vi "PECT - Scan.vi"() -> ()   [LabVIEW 2012]
uses:
  <vilib>/DAQmx/write.llb/DAQmx Write (Analog 1D Wfm NChan NSamp).vi
  <vilib>/DAQmx/read.llb/DAQmx Read (Analog 1D DBL 1Chan NSamp).vi
  <vilib>/DAQmx/read.llb/DAQmx Read (Analog Wfm 1Chan NSamp).vi
  <vilib>/Instr/_visa.llb/VISA Configure Serial Port (Instr).vi
  <vilib>/DAQmx/create/channels.llb/DAQmx Create Channel (AI-Voltage-Basic).vi
  <vilib>/DAQmx/configure/timing.llb/DAQmx Timing (Sample Clock).vi
  <vilib>/DAQmx/configure/task.llb/DAQmx Configure Logging (TDMS).vi
  <vilib>/DAQmx/configure/trigger.llb/DAQmx Start Trigger (Digital Edge).vi
  <vilib>/DAQmx/create/channels.llb/DAQmx Create Channel (AO-Voltage-Basic).vi
  <vilib>/DAQmx/miscellaneous.llb/DAQmx Fill In Error Info.vi
  Global_data.vi
  <vilib>/express/express analysis/Spectral/Block/exnSpectralBlock spectral measurements PSD poly.vi
  <vilib>/express/express analysis/Spectral/Block/exnSpectralBlock spectral measurements PSD WFM.vi
  <vilib>/express/express analysis/Spectral/XNode/ExpressSpectralMeasurementsBlockNode.xnode
  <resource>/objmgr/daqmx.rc
  <vilib>/measure/NI_MABase.lvlib
  <vilib>/Platform/NI_3dgraph.lvlib
panel:
  in  "Backward scan":bool
  in  "X-length count":dbl=20.0
  out "No.data":i32
  in  "Save Scan mode":bool caption="Save Process"
  in  "Plot style":i32(ring)=5 items=["cwLine"=1, "cwPoint"=2, "cwLinePoint"=3, "cwHiddenLine"=4, "cwSurface"=5, "cwSurfaceLine"=6, "cwSurfaceNormal"=7, "cwContourLine"=8, "cwSurfaceContour"=9]
  in  "Stop 4":bool
  in  "Forward scan":bool
  in  "ViewMode":i32(ring) items=["cwViewXYPlane", "cwViewXZPlane", "cwViewYZPlane", "cwViewUserDefined"]
  in  "Stop Scan 2":bool
  in  "Emergency Stop":bool
  in  "Stop 3":bool
  in  "Home Y":bool
  in  "Home X":bool
  in  "Back":bool
  in  "Front":bool
  in  "Left":bool
  in  "Right":bool
  in  "Stop Scan":bool
  in  "Move Distance (mm)":dbl=10.0
  in  "Scan":bool
  in  "Pulser Trigger Source":tag="/Dev4/PFI1" caption="소스"
  in  "Open":bool
  in  "Tab Control 2":T1(tab)
  out "Hall sensors signal":waveform(dbl)[](graph)=[{"t0"=timestamp(3525645621.636764 s since 1904-01-01), "dt"=1.9999999999999944e-06, "Y"=array[2100 elements], "attributes"=variant("NI_ChannelName"=variant(string "Dev1/ai0"), "NI_UnitDescription"=variant(string "Volts"))}, {"t0"=timestamp(3525645621.636764 s since 1904-01-01), "dt"=1.9999999999999944e-06, "Y"=array[2100 elements], "attributes"=variant("NI_ChannelName"=variant(string "Dev1/ai0"), "NI_UnitDescription"=variant(string "Volts"))}]
  out "Feature Extraction":dbl(graph)=0.021153968958947764
  out "Waveform Graph 2":waveform(dbl)[](graph)=[{"t0"=timestamp(0 s since 1904-01-01), "dt"=1.25e-06, "Y"=array[8000 elements]}]
  out "Power spectral density":cluster{"f0":dbl, "df":dbl, "magnitude":dbl[]}[](graph)=[{"f0"=0.0, "df"=238.09523809523876, "magnitude"=[-25.4340272409559, -28.495970805276507, -69.09064054555873, -79.11355871279994, -75.69366097931027, -84.18131507822396, -80.50168881348966, -82.72314293089615, -87.19630499623688, -82.83568021481967, -89.95290866002237, -85.90392585035596, -87.41269111550386, -91.40893948681482, -86.69370819914215, -93.36336146616782, -89.019380476413, -89.73232030153878, -94.58261196624535, -89.16287927388944, -94.965890302584, -91.86846413178648, -91.95327957161693, -97.62687167891286, -91.59993648735762, -97.30685711015555, -93.8350762480425, -93.27921214218685, -99.59438563802183, -93.1824258709588, -98.3113125531512, -95.45425138584356, -94.39327135467576, -100.65352961491782, -94.55889081970952, -99.40788907105079, -97.93617495318924, -96.19517579047603, -103.97036797797732, -96.40295202889732, -99.7036956909043, -99.48760137175819, -97.46192979187015, -106.29271483151813, -97.51447379981207, -99.86179280251669, -100.43811038443037, -97.59011642740829, -105.58363666166275, -99.01126121197593, -101.01575323613292, -101.90167607549864, -98.61952569586691, -106.73670466995647, -99.29976101634999, -101.54959604687718, -105.17330050767885, -100.09392305285375, -109.78264848704497, -100.98914236173123, -101.81665207962125, -105.42358374403365, -99.82880728595141, -107.07330885402075, -101.07712607444097, -101.03780825357597, -107.32811151840846, -101.221643458408, -105.63776326231454, -101.8420593566944, -101.80081629073969, -107.47915505307212, -101.12986632760553, -106.84901404755908, -102.73715610491038, -101.51552854007832, -107.28771371003282, -101.3928633472346, -107.44515355816633, -104.89304864643535, -103.1455098860718, -110.19910428997925, -102.73063833081197, -107.57101838377707, -104.90574568581201, -103.72599931018533, -109.97178587260123, -103.24611921258705, -108.36098023558972, -106.6408311450923, -104.73569536588386, -116.21683530762306, -105.02627439976544, -107.15856030450797, -109.81191038702062, -105.53476822084077, -119.10077766590356, -105.31867536160968, -106.9718410299748, -108.34458911268797, -104.70307996109247, -114.76704583683203, -106.29948298493936, -108.55077108437321, -112.16618350190343, -105.98453547558171, -114.68576835450673, -107.50968901677987, -107.89174277914348, -111.59875709602721, -106.69368240333122, -114.93273233954758, -105.23904516482949, -106.00272331017348, -110.36103151258544, -104.93177986717492, -110.8835476773746, -106.69346348818806, -106.66103973993782, -119.11729839814336, -108.06338160849775, -114.5879267769655, -108.59816838472844, -107.53189260743514, -114.07390818184973, -106.70996756049796, -113.27381274118753, -109.50270539577696, -107.37282420343303, -113.4779718725949, -106.04267666963091, -111.30294425571472, -112.46717993668915, -109.13164915488709, -116.65287200885172, -107.03002573045511, -110.21479040603631, -112.476075561056, -106.97710947409149, -119.42145279296255, -108.3200486628316, -110.46641858585929, -117.16650627564961, -109.73297826697552, -120.31689830731365, -107.19513745371916, -110.66663569403087, -113.30365980039964, -110.01971553524372, -123.68660617105166, -110.8171755739396, -111.11382172813546, -117.76239209582961, -109.49899370205401, -115.22252846498625, -111.1932077339224, -112.38235939086871, -118.22207022901702, -110.6546796895719, -116.97450780644367, -110.82401674194465, -111.96705198878843, -118.28092956599232, -110.5621503678909, -121.25720613496851, -111.98371482341479, -113.27928013246557, -111.96833712758355, -108.56859286664552, -120.32790468431601, -110.82699792221703, -110.79062667340345, -122.65756767769517, -110.48843456045427, -116.8782055296399, -115.43719816168479, -114.47619780315773, -121.42183196132746, -111.60631415727042, -120.68077308056417, -109.35478690141552, -109.03210709352732, -120.6260555904793, -109.47936424950136, -113.33719701518146, -112.88325992990137, -110.99901978536154, -123.19636626521421, -109.09861317900774, -113.33125158106256, -115.35673297389727, -112.77249677632989, -124.61163141716472, -114.68140920359865, -121.89642913325117, -115.47413298424323, -112.82196063671608, -127.87542521315149, -111.54178118788309, -113.6448752704395, -120.76569423868874, -112.98651214877823, -123.18868565400437, -115.41399838634062, -115.46853076016815, -116.40989072804102, -110.69611347288615, -132.23164080331392, -114.76376391429793, -121.7246597336247, -117.46893009589195, -114.01899156779395, -125.22079066032327, -114.59524199183258, -114.50034890537415, -122.9532092227648, -113.72727798159212, -125.65163915514907, -113.4793801211504, -110.4090756414644, -125.63592649005872, -114.22938378193007, -116.74947251106808, -121.60535557984142, -116.79385283402802, -122.44667696630361, -113.43873413563811, -123.28159708694415, -113.92892974938164, -114.01193823589753, -121.62751955742443, -118.76839573694522, -125.52998605097204, -115.19609643487229, -117.49409595176479, -117.08423885198002, -119.48314867245172, -125.01675515413412, -117.92668164142911, -115.55962389856793, -125.63488616674975, -119.11862859365166, -114.78860770332909, -117.18339781294443, -111.18063004722558, -118.31775966044624, -111.6867367949252, -114.57226159377, -119.36541212960576, -113.90245139442648, -132.46343443313128, -120.1282759002165, -121.05279009698619, -118.9115822659523, -121.23280439248342, -116.31914159559688, -127.38829313950257, -117.34673005740623, -115.95249861902771, -114.9301657394146, -123.22361802797445, -110.83274939062106, -116.16624248562111, -116.76753364192771, -113.94454545069023, -122.95736945775944, -118.66755800656253, -129.1462641201204, -116.6351050110328, -117.22529407303742, -123.80212197360244, -115.89792176423389, -114.25823938606595, -125.60467961977515, -114.59958849364433, -121.70071005514421, -118.25968972451209, -114.69929400946009, -123.88209034116528, -115.03869272537257, -117.52034211782204, -115.27990843516797, -117.85366603932033, -125.16865559622727, -118.21960424638507, -119.69008755413566, -117.24640963460672, -114.32867295013791, -119.1576982419508, -122.85495988425586, -116.3373010103401, -114.53730203699834, -115.67017599990201, -127.144321037601, -115.73849102686786, -117.7626163106355, -119.7346592991025, -117.41317517684553, -125.0417974461613, -114.5488949833583, -116.59812516173781, -119.91064563147799, -115.27933218667663, -122.09990513751134, -120.95678574143693, -123.25641714743752, -112.5173710452192, -113.53735878806998, -129.23914933506734, -116.27157269711533, -148.4020512032711, -118.84888216023774, -123.82550527215588, -116.87770979616658, -111.32191810025745, -124.32675905891588, -114.37182733794062, -121.10713785851372, -122.59698730059695, -116.38346694563282, -121.69144349152856, -119.00883142493832, -110.81886738196273, -120.7909830607913, -115.01780448665316, -114.52055121633796, -132.6824191654361, -116.330695115645, -126.4664151018508, -118.32717907779282, -118.7288071595281, -120.42749846140066, -112.53185615773879, -124.26026008984286, -114.24089252048742, -120.00368190003405, -114.71738500842926, -112.92262025927133, -129.21127897188563, -113.5947811765517, -117.80802009651353, -117.0133790103226, -112.19210322760304, -118.17549968071762, -119.3256187825503, -118.84981507334446, -121.39118969751144, -114.64543555194373, -119.84814933224528, -114.09123407848944, -116.22899352170892, -116.41650104077173, -113.70057202673476, -124.52773908304957, -114.87372641784933, -116.11651108221098, -121.68680962246994, -115.78306007961302, -122.22621008657796, -118.81157995182392, -113.9402115821658, -132.636729517989, -114.49554876936634, -119.50980190398928, -123.27410972236837, -118.52851881066383, -122.25212982572599, -117.13947036230024, -120.85005588797962, -118.41526503460501, -117.61788553858068, -126.3872056783977, -114.98198608543298, -119.7789938911847, -120.84873579392627, -114.38831474301695, -153.35954756825245, -113.19505610638078, -114.17454820985151, -127.41069917723112, -114.92677241657191, -125.49053973810628, -113.36382196587914, -119.96785250843519, -122.47388530423243, -116.38671253508838, -120.0905790211523, -119.83326265062107, -117.88168146696918, -122.3132169880757, -115.87324909105399, -125.92003267803432, -113.96860176867415, -114.49156118371398, -127.52634390035722, -115.05967156528004, -126.82020221981517, -117.93643187259194, -116.51163213641807, -119.47551219110167, -119.55225172256931, -116.9512257852571, -122.23153124485954, -120.8368476753637, -121.48473913072222, -115.83122660909913, -135.74260014140523, -116.58358375805423, -118.15236945484727, -119.06674062398864, -115.7844834762477, -125.06111738611818, -114.7801535050972, -115.2696605691888, -123.98656374010793, -119.29025555731172, -118.29146803784099, -119.55696172158135, -118.06884171238352, -127.81587648134607, -120.41730580797976, -123.49626136731604, -112.2147141798107, -116.22555232584983, -132.79419178871254, -119.66964883124663, -117.20946469243259, -118.20939292735417, -115.6951914646649, -129.64892855822356, -114.27056999288617, -120.31005512957381, -117.41846777372632, -115.50158386260813, -124.69777160737624, -115.2892897247205, -123.61522771666871, -113.75248734362687, -113.22999749252833, -129.3490509395313, -116.88137735661701, -116.94110280242681, -119.50244079984806, -119.30521139999144, -128.17199984115797, -118.06736594940236, -116.05331575995922, -121.29670750650897, -116.1140297602044, -125.090619084802, -121.41807296062154, -120.01332757902264, -120.54914530643151, -116.49738633175463, -122.32551291835904, -118.3190808346865, -118.92638453656723, -122.48819531011718, -117.01021725424317, -120.98896352560598, -117.23831688685218, -121.27915259197124, -121.20017251921661, -117.6155648860373, -120.91300272912063, -117.94438460863424, -115.94437430101533, -123.35904829443987, -117.74011174503076, -121.54935745388448, -120.82564553545025, -121.98951430455743, -120.24858103448778, -116.44403527138395, -112.79571494351876, -112.42801913096545, -110.1697573019791, -115.34500457736401, -119.81921052956707, -129.82600951154313, -115.5862301263047, -112.59292882433087, -120.79009137478283, -131.32849293387295, -113.61194478398238, -123.48568856527031, -119.17507777781304, -123.09261867490484, -116.97755217417308, -123.94453461434183, -116.58080525616379, -119.64289646280756, -122.90202645580743, -126.66219093058154, -121.95048829056148, -115.72578023509817, -116.70117814464484, -121.91050280869723, -118.25299095698178, -116.45905559047064, -132.57794493731578, -121.65327820443292, -120.9816664775787, -117.17270262269045, -120.27433984830965, -125.89418976028173, -119.09563505847817, -126.9693215534833, -113.17465524665704, -118.98702092883116, -119.83822568580342, -120.45832738089722, -120.67735960513633, -127.38676010839353, -127.65777338183055, -118.37446329057411, -115.61355494839711, -119.94568688114103, -116.06619937633681, -126.348857777089, -118.92850079147068, -119.5416617639739, -132.47075644221843, -118.08809356028496, -123.16186463092723, -121.51579486791232, -122.88983670053283, -129.5195538417256, -120.4730389608841, -132.16486858341602, -122.34690358436781, -120.71922104337597, -114.29260860841114, -117.67902631803368, -124.7040155514909, -123.51274592117205, -120.02297921674332, -136.54655493811157, -120.45629227407751, -119.06410204276258, -127.91681714792554, -122.82090055753153, -125.16838176650813, -121.79565386970478, -119.79607311590995, -126.54861375039647, -121.59135878113302, -132.8348640697562, -118.1305434733294, -120.46070148841905, -122.69571910896963, -117.6534954653865, -124.15742546824006, -120.73646926947502, -124.82696993800742, -124.513836786494, -123.15395713389651, -124.62395468806395, -117.21365768658171, -119.32635871968456, -121.48532284413152, -119.38242892643675, -126.25575652510352, -123.27133124029851, -117.58533922728374, -118.17710108929799, -114.99496360200965, -117.77133194647278, -111.34898201101595, -111.50817058307922, -119.0703124690998, -127.70676079885351, -121.8704969141074, -125.93154214283446, -118.65628450081473, -122.47918878348962, -117.9651589546518, -126.13560583004508, -122.42294805637847, -133.924453763793, -117.2082573038767, -117.6525335446734, -122.92077297426977, -122.04624645756786, -116.43289028226238, -117.93180959338378, -129.02356734231915, -117.95493621286326, -120.7555929766252, -120.76782849311112, -123.06287498470708, -117.83798593857965, -123.43423215434719, -120.15190119516652, -120.48240443128407, -143.29738987393452, -123.46572247444769, -120.89055325172792, -125.66715973809033, -118.26887578998644, -117.01836200028421, -121.33021830755509, -119.68846363313813, -122.60689066103069, -116.26858138914181, -119.59360791972998, -122.94866175463353, -114.174409515556, -118.00516930888391, -121.56978543579633, -135.87799017759036, -117.50816594504829, -122.82539428457626, -123.82103443155845, -124.77975840345442, -121.13340798086698, -120.93607435603558, -133.15787160745222, -120.70545628137863, -125.02155972441679, -122.04666465472178, -118.01234649746348, -127.88767491042842, -119.02096620167217, -120.16031065152875, -122.25406107859625, -121.72733059051095, -120.61357375519918, -118.63962847172827, -134.3857741605498, -116.3600853185034, -117.26695700691671, -119.9176982185873, -113.45576465218444, -126.69779573632724, -114.39554522802246, -116.8457146515868, -116.34219889483086, -119.30011291548334, -120.01163291843496, -114.29497178248809, -127.65687642749229, -119.58556923753022, -129.8593054181261, -122.2353645100479, -120.79536520223796, -119.83284028355028, -117.7991246185715, -128.390292904734, -119.78079925213122, -125.478913448993, -113.89747777944768, -112.66620124153357, -124.3475049842711, -120.85847303094337, -132.91807981902295, -119.523494985723, -116.65149909866443, -119.73287290436721, -127.63237851524192, -127.23413304048789, -120.87585453904362, -121.08540368080186, -134.91071939669257, -117.75375801669338, -117.2683014590723, -120.9739099492833, -118.23809733632451, -120.94065804928206, -123.88077510875804, -118.13812819300607, -122.60294123365466, -126.97075898006995, -120.18754789731035, -124.71238663441227, -120.55456557278582, -130.94599087480253, -111.18288669417035, -112.27708791831247, -126.0512034600378, -117.41881712783596, -128.20553880273903, -117.29482600885808, -118.2045526390752, -127.81966672699878, -117.03716165902529, -115.46711739757512, -117.15363929234843, -121.87599671671335, -121.19736800869221, -126.5301786755875, -131.20754947382918, -124.40138004810741, -129.0562496906515, -121.06816554587536, -121.01023627802867, -138.6137911215848, -120.12495002524031, -121.38510517514229, -122.79804220535513, -116.97501378195477, -118.82011581137473, -114.0229185604644, -119.54287501990726, -114.64474566771625, -117.76935669872461, -123.81082574158907, -118.51678358865587, -128.9664755188374, -123.45357998434133, -122.74888841574231, -120.74640581234044, -126.956344345126, -119.95682140104577, -118.8873101779055, -124.41062359284174, -128.97304498664363, -123.86287113204068, -127.30257087528216, -120.61364220528216, -114.45119129304715, -119.68384044686806, -131.29639185291157, -122.31250766293485, -119.57420865241102, -124.74014026002448, -124.87593035709094, -118.4566565612952, -123.76236085976001, -120.84780538841838, -117.68987599773281, -135.06195695255914, -122.56143585795171, -129.04610316842883, -118.32313199570537, -117.77093802786419, -124.46572845786741, -129.1123298336903, -120.88470269965448, -116.69988985752187, -116.84054667499878, -133.76883696987278, -122.32434984927302, -124.98940594457933, -122.56515592789917, -118.31562562243366, -133.97049179545627, -122.33220627999802, -131.16753675316977, -124.69828063969263, -116.37621154460467, -126.1833423168025, -129.62937634161355, -118.46241371150788, -117.52851478852457, -125.32425037236442, -119.0327364293772, -124.2861355894013, -123.24573502278234, -125.52155812053758, -113.75743410709823, -114.79513162658353, -128.58142362588052, -122.48277095196701, -118.94747544412269, -123.86988127835491, -124.78140456983323, -121.53998481875398, -116.01432822539552, -119.20174681160661, -122.75167725800814, -120.58657749420254, -118.51141061842183, -119.24457006171983, -131.43641234223372, -116.00759139055087, -121.24442216102587, -123.29371279953725, -117.608355420454, -116.33684374617326, -118.06291688281922, -121.88761866022774, -121.54820313120047, -119.5051369873635, -126.56611158390913, -118.84012713615805, -121.09285296522563, -124.67955377692547, -147.31451139022337, -116.80660421066897, -114.8367853755961, -120.41026468628925, -123.65666101895222, -119.64837119787269, -116.77480172559095, -116.54263359173909, -124.75286620868079, -117.33721912698883, -116.51795620907136, -118.50086748176733, -128.10381328920522, -122.78098994574157, -120.24716756092855, -119.52743204722819, -115.00407387659232, -108.2853711552629, -108.61086943894702, -119.6228894146785, -124.11132022420912, -125.6202218409766, -123.1749360787656, -118.1971196161698, -123.95075368058998, -121.72140109898365, -123.27106899042522, -123.73035629887062, -121.24369679109273, -121.07381526465288, -113.13965659723667, -118.330755475899, -118.40249076804484, -111.59630598649044, -116.1569506845575, -125.67326089915758, -125.85723567111906, -119.24293277595024, -117.87067617433537, -120.70936924059559, -131.8090588468898, -132.98711569625004, -123.63274249467587, -122.75476917502559, -126.12873814250243, -120.53144270605179, -129.07030822919336, -122.7889410422919, -124.35405971166259, -119.63968579420454, -139.0154441054289, -129.47962001806934, -121.86548015410847, -128.6818469257012, -121.40195873232601, -138.64231053781285, -124.22025721762265, -124.06073958736941, -126.71929802352521, -131.7498459276443, -120.68144109742178, -122.6325588818875, -126.80796617875095, -124.92487955227033, -136.94498040498806, -124.26704334219014, -123.21376211221711, -140.25352033075964, -129.53222319772195, -122.58541579060463, -122.1996729592375, -125.66642108013673, -125.66310429236694, -120.09682773706965, -125.27326633941439, -121.55721878725502, -121.22507119941083, -121.53716878624485, -136.20685498111987, -128.15260146013156, -120.03473972471616, -124.60755958763912, -124.73082500077143, -123.93425949983688, -131.04483249265184, -121.7957035014449, -127.09321441816094, -133.6144579272493, -124.69014595896968, -130.4902091211609, -121.18031440773905, -128.00033943961677, -125.88991118115149, -118.865310745079, -123.69668867733147, -117.98756965862728, -114.40013091842827, -118.28685032521078, -122.23464196869948, -124.8440422629961, -129.66281606870848, -119.440534215621, -124.54391783563877, -124.93447967158188, -121.7258558761523, -122.28817885403082, -127.06889620458577, -128.92172974939206, -120.62932166634072, -126.06847321900452, -123.31471168429935, -121.80350826545656, -129.2574604322076, -125.67225933193998, -125.7801671825605, -129.53804733161627, -119.56756644124712, -128.82490314699373, -124.7689736295626, -120.50019729114693, -124.50603158563972, -122.8120627011088, -125.60528875555717, -123.8817354922713, -124.05570537836674, -120.94568834491936, -118.06056028605255, -124.24390361274648, -125.5716703018188, -127.71949519914061, -130.7001652968252, -126.27701412017494, -133.76810134709916, -128.4738939614179, -120.302550881701, -118.91298143662928, -124.9077318110765, -127.16253699189492, -118.11405934812818, -117.52028071290711, -140.95620572748925, -123.61977932545628, -131.0334379970501, -125.88948384968432, -127.81552331993379, -121.92316280719056, -119.05911238768732, -126.83773251459189, -123.52627415002164, -120.8779561023192, -123.66683567603742, -131.64300993967345, -123.62895847772963, -116.89792951363142, -120.1068259250195, -117.92484706459337, -115.58208487778379, -120.76803581628594, -123.95408562090736, -122.79456549632754, -134.5305398779298, -123.57040300991032, -128.40634159414552, -123.70102187824159, -118.24970739397313, -119.66483900349026, -127.78024313111393, -120.3547204111785, -125.49305364308705, -119.49505591004302, -120.50920386196539, -119.03509516851003, -114.24667300009652, -121.60538636584391, -119.95304417598024, -122.24585853682832, -128.63653016912684, -116.04810628805795, -121.94159862131235, -122.59928204398939, -121.4532410501923, -128.6511474663462, -130.83715595958148, -121.71998300574741, -116.91426629511156, -113.587592058512, -115.59736707638731, -124.65300822631244, -133.32538684258748, -124.02289142873636, -121.54278890993639, -119.02596809402394, -108.90572887117857, -112.14974069608851, -129.21149299565423, -118.82148342951197, -116.65510894288538, -118.39609618084175, -116.53502642884725, -122.47549439965209, -122.23125657046063, -123.68081343116663, -120.67915071600007, -123.6899360128769, -118.56721985209728, -118.36641581191942, -126.96724630704657, -119.36877661672403, -123.07698921198843, -117.80772421906035, -122.82545076270567, -118.82755071380888, -117.21030132539394, -129.760567864525, -118.0816708063509, -125.80573274113647, -121.18434666182338, -121.80987210832065, -130.99259828357094, -125.47223579895922, -123.86818606677002, -118.7118158196511, -119.27778317338742, -127.27333258839096, -119.90672352079164, -140.78772370844268, -118.08251080057329, -119.86636232122572, -118.69482489738232, -119.19106512767372, -123.70988914879189, -121.92566832147995, -123.41378261726373, -120.1715186070818, -117.9079629421116, -117.41960207545632, -123.72833996166874, -127.24377206607298, -124.99098647980887, -129.48803701799955, -129.92351350561592, -120.79284154834647, -119.29601975194524, -136.17244775530037, -126.73975437546255, -128.84068276143336, -125.66374985701982, -136.69026010435715, -125.44409235146617, -119.28138070315057, -118.65017329869724, -118.02521532826772, -122.23736063759657, -121.27846943548622, -116.69850478126861, -119.7711336696722, -123.70776561180185, -118.43344549561263, -123.92390877157247, -117.19637143066551, -117.64112988205311, -127.78399195238529]}, ...(2 in all)]
  in  "3D Surface":refnum<k7>(container)
  out "Feature Extraction 2":dbl(graph)=0.021153968958947764
  in  "Tab Control":T2(tab)
  in  "X-length":dbl=20.0
  in  "Step X":dbl=0.2
  in  "COM Port":refnum<visa-resource-name>="COM4"
  in  "Baud Rate":u32=9600
  in  "Data bits":u16=8 min=5 max=8 step=1
  in  "stop bits":u16(ring)=10 items=["1.0"=10, "1.5"=15, "2.0"=20]
  in  "Parity":u16(ring) items=["None", "Odd", "Even", "Mark", "Space"]
  in  "1 Min":dbl=0.4
  in  "2 Max":dbl=6.0
  in  "1  Max":dbl=6.0
  in  "2 Min":dbl=0.4
  in  "Y-length":dbl=20.0
  in  "Step Y":dbl=0.2
  in  "1 Rate":dbl=0.2
  in  "2 Rate":dbl=0.4
  in  "Travel per Pulse (mm)":dbl=0.002
  in  "Cur. Pos X":dbl=-33.28 format="%#.4f"
  in  "Cur. Pos Y":dbl=30.0 format="%#.4f"
  in  "Save Speed":bool
  out "Move X":bool
  out "Sample per Channel AI":dbl
  out "Sample per Channel AO":dbl
  in  "Pulser Cycles":i32=10
  in  "Logging Mode":i32(ring)=10231 items=["Off"=10231, "Log and Read"=15842]
  out "Actual Sample Rate":dbl=500000.0 format="%0.2f"
  in  "Physical Channel":tag="Dev4/ai0"
  in  "Min Voltage":dbl=-10.0
  in  "Max Voltage":dbl=10.0
  in  "Terminal Configuration":i32(ring)=10083 items=["default"=-1, "RSE"=10083, "NRSE"=10078, "Differential"=10106, "Pseudodifferential"=12529]
  in  "Sample Clock Source 2":tag="OnboardClock"
  in  "Sample Rate":dbl=500000.0
  in  "TDMS File Path":path
  out "Actual Sample Rate 2":dbl=800000.0 format="%0.2f"
  in  "Physical Channel(s)":tag="Dev4/ao1"
  in  "Min Voltage 2":dbl=-10.0
  in  "Max Voltage 2":dbl=10.0
  in  "Sample Clock Source":tag="OnboardClock"
  in  "Sample Rate 2":dbl=800000.0
  in  "Offset":bool
  in  "2 Plots":bool
  in  "Edge":i32(ring)=10280 items=["Rising"=10280, "Falling"=10171]
  in  "Digital Trigger Source":tag="/Dev4/PFI0"
  in  "Duty cycle %":dbl=50.0 format="%#.2f"
  in  "Output Array":T3(array[cluster])=[{"Waveform Type"=2, "Amplitude"=10.0, "Frequency"=300.0}] {"Frequency" format="%0.2p"; "Amplitude" format="%0.2p"; "Waveform Type" items=["Sine Wave", "Triangle Wave", "Square Wave", "Sawtooth Wave"]}
  # "Pulse Shape"
  # "Trigger Settings"
  # "Data Processing"
  # "Pulse"
  # "Hall Sensors Signal"
  # "Feature Extraction"
  # "Power Spectal Density"
  # "COM  Setting"
  # "Speed  Setting"
  # "Scan  Setting"
  # "Pulse  Channel"
  # "Pulse  Timming"
  # "Sensor  Channel"
  # "DAQ Timming"
  # "Logging Settings"
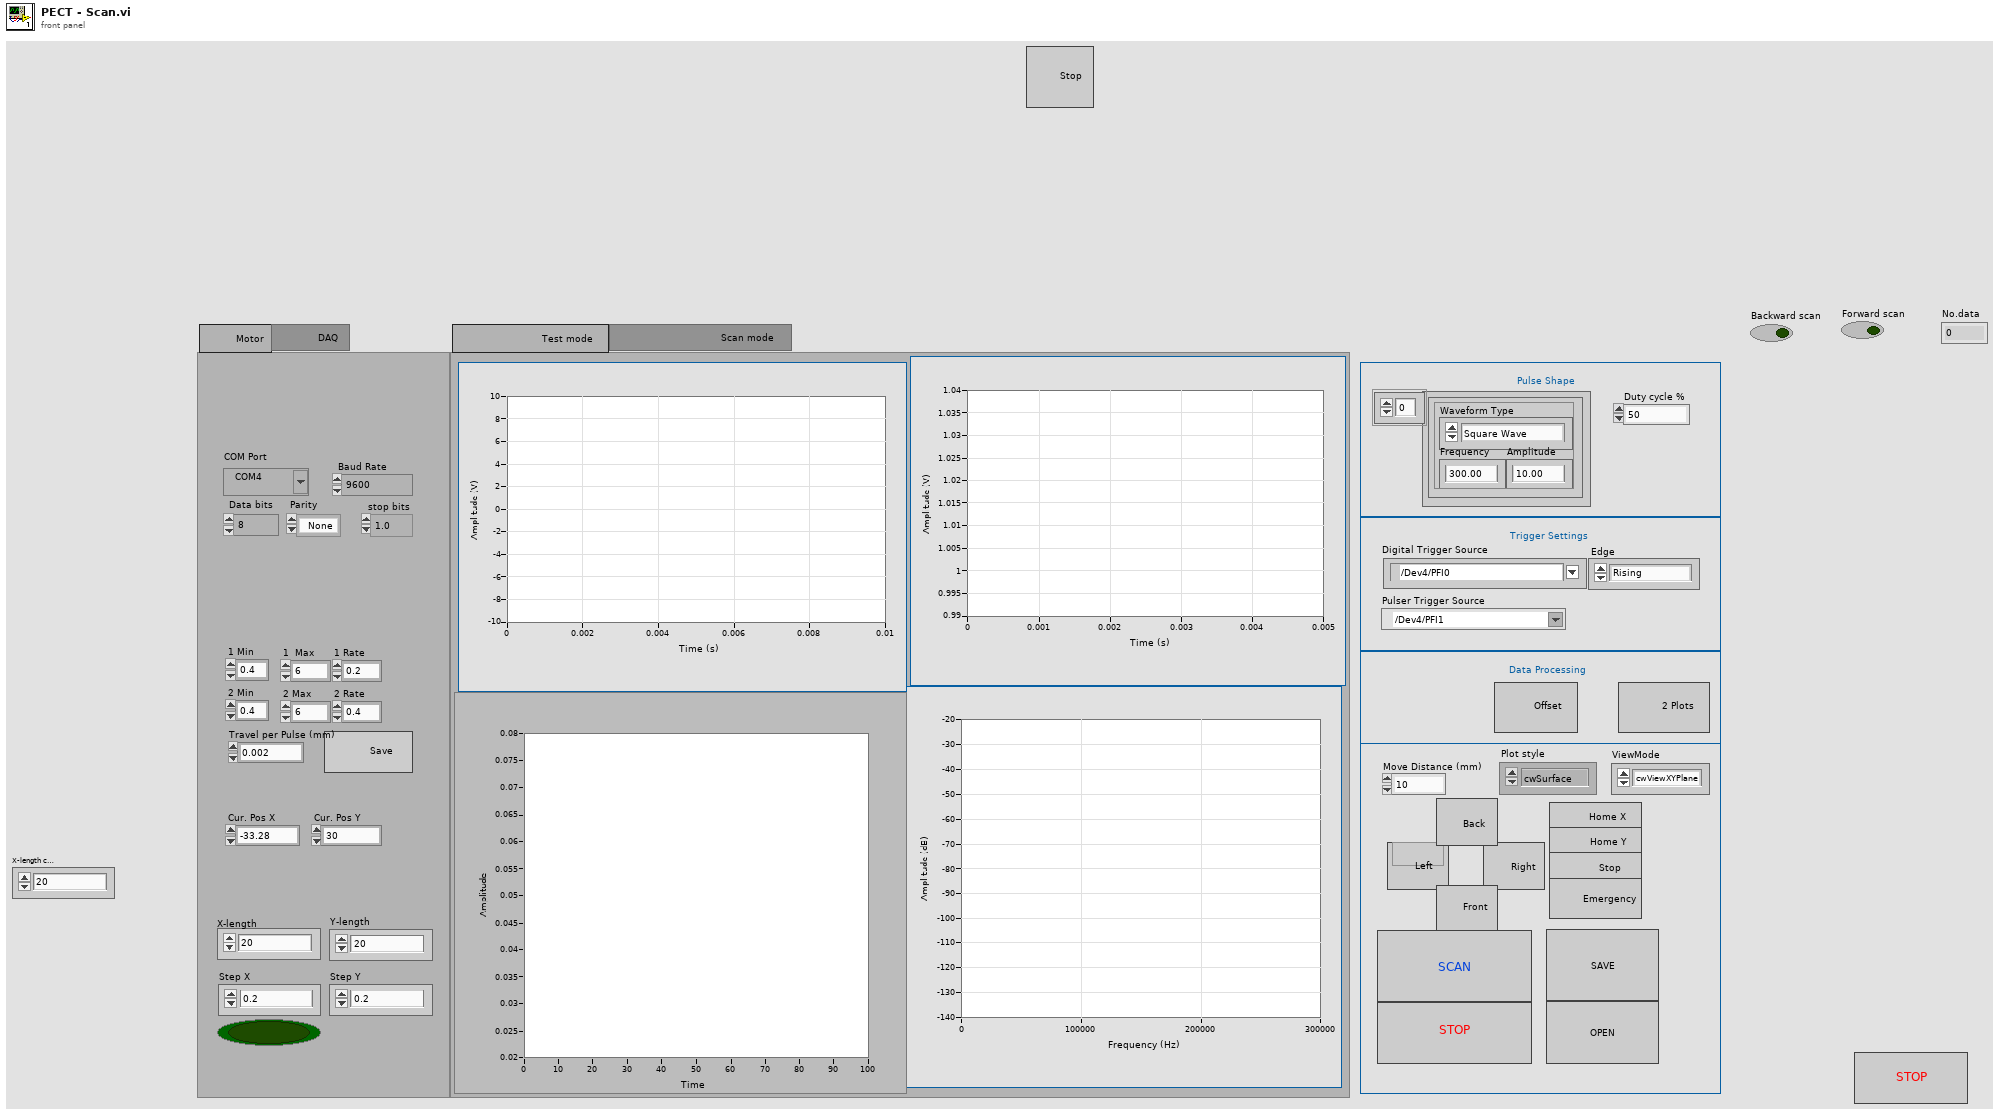
[diagram p1: front panel]
types:
  T1 = enum32{"                    Test mode                   ", "                          Scan mode                      "}
  T2 = enum32{"        Motor      ", "          DAQ        "}
  T3 = cluster{"Waveform Type":u16, "Amplitude":dbl, "Frequency":dbl}[]
  T4 = cluster{"Waveform Type":u16, "Amplitude":dbl, "Frequency":dbl}
  T5 = cluster{"averaging mode":u16, "weighting mode":u16, "number of averages":u32}
  T6 = cluster{"dB On (F)":bool, "unwrap phase (F)":bool, "convert to degree (F)":bool}
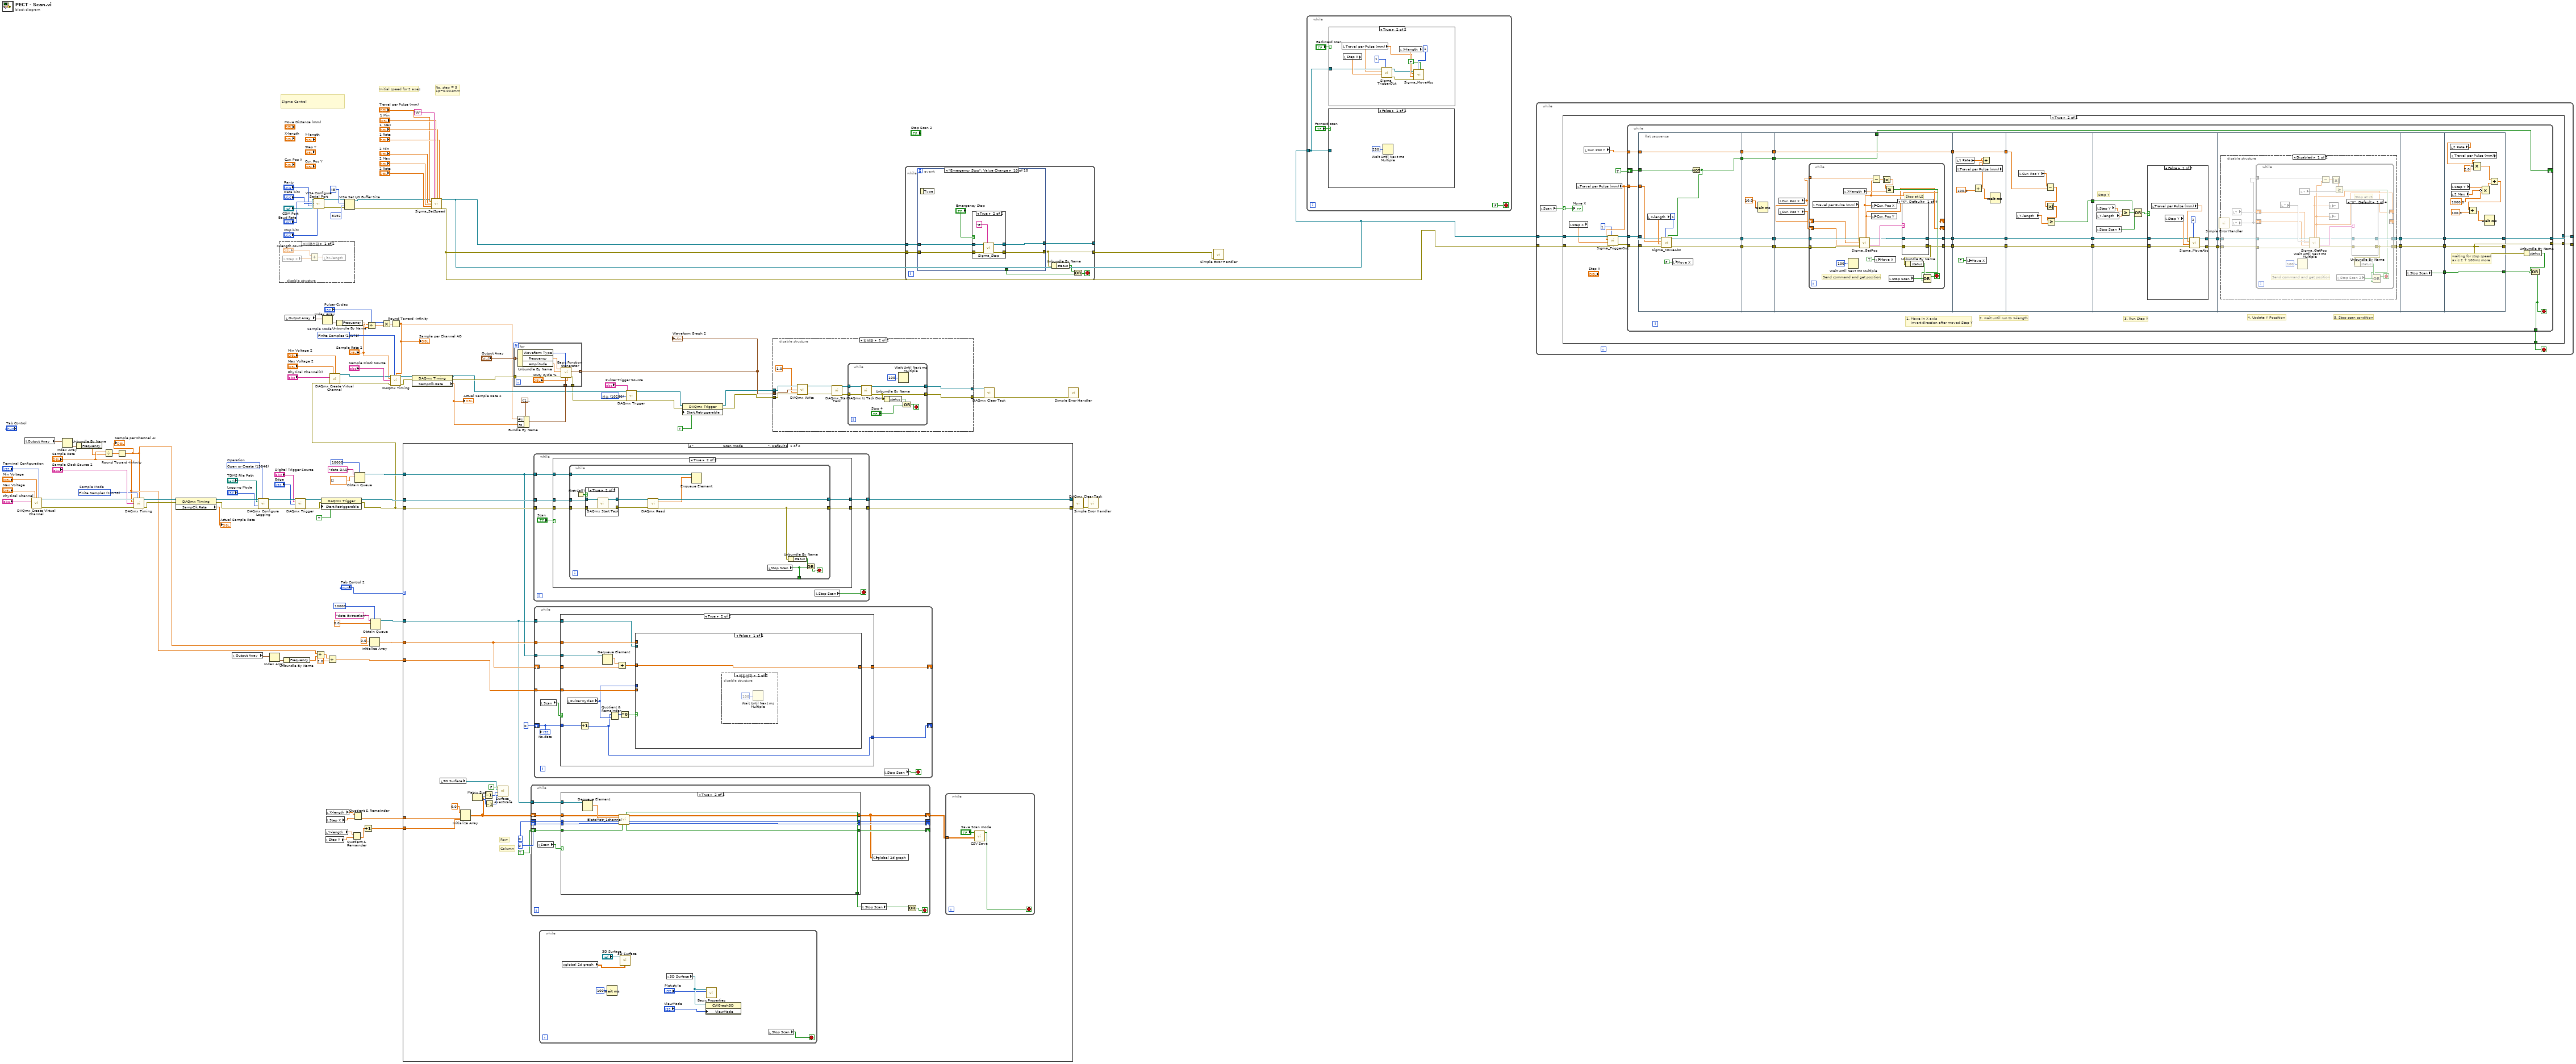
[diagram p0: block diagram]
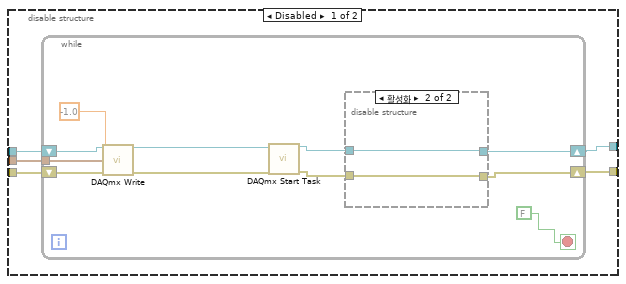
[diagram p3: hidden frame]
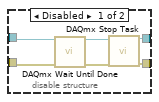
[diagram p4: hidden frame]
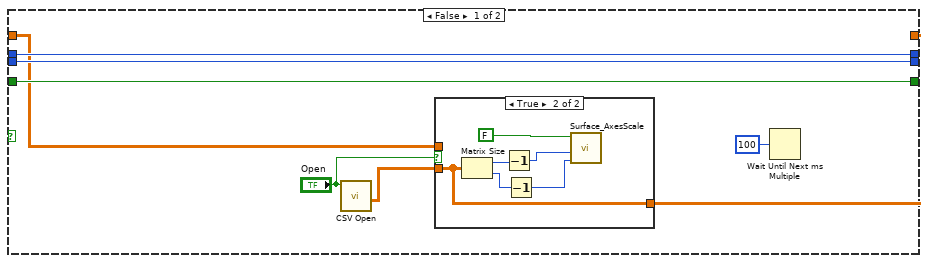
[diagram p5: hidden frame]
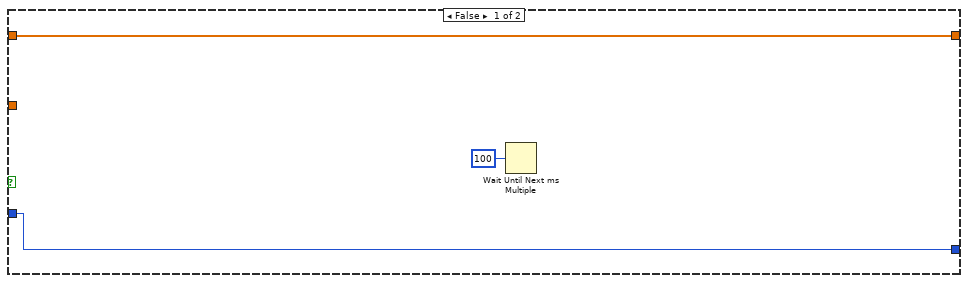
[diagram p9: hidden frame]
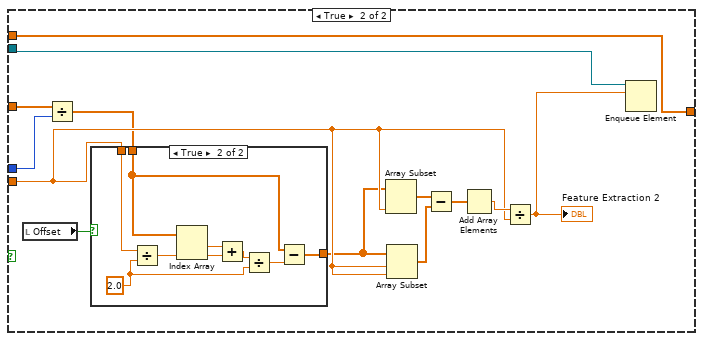
[diagram p11: hidden frame]
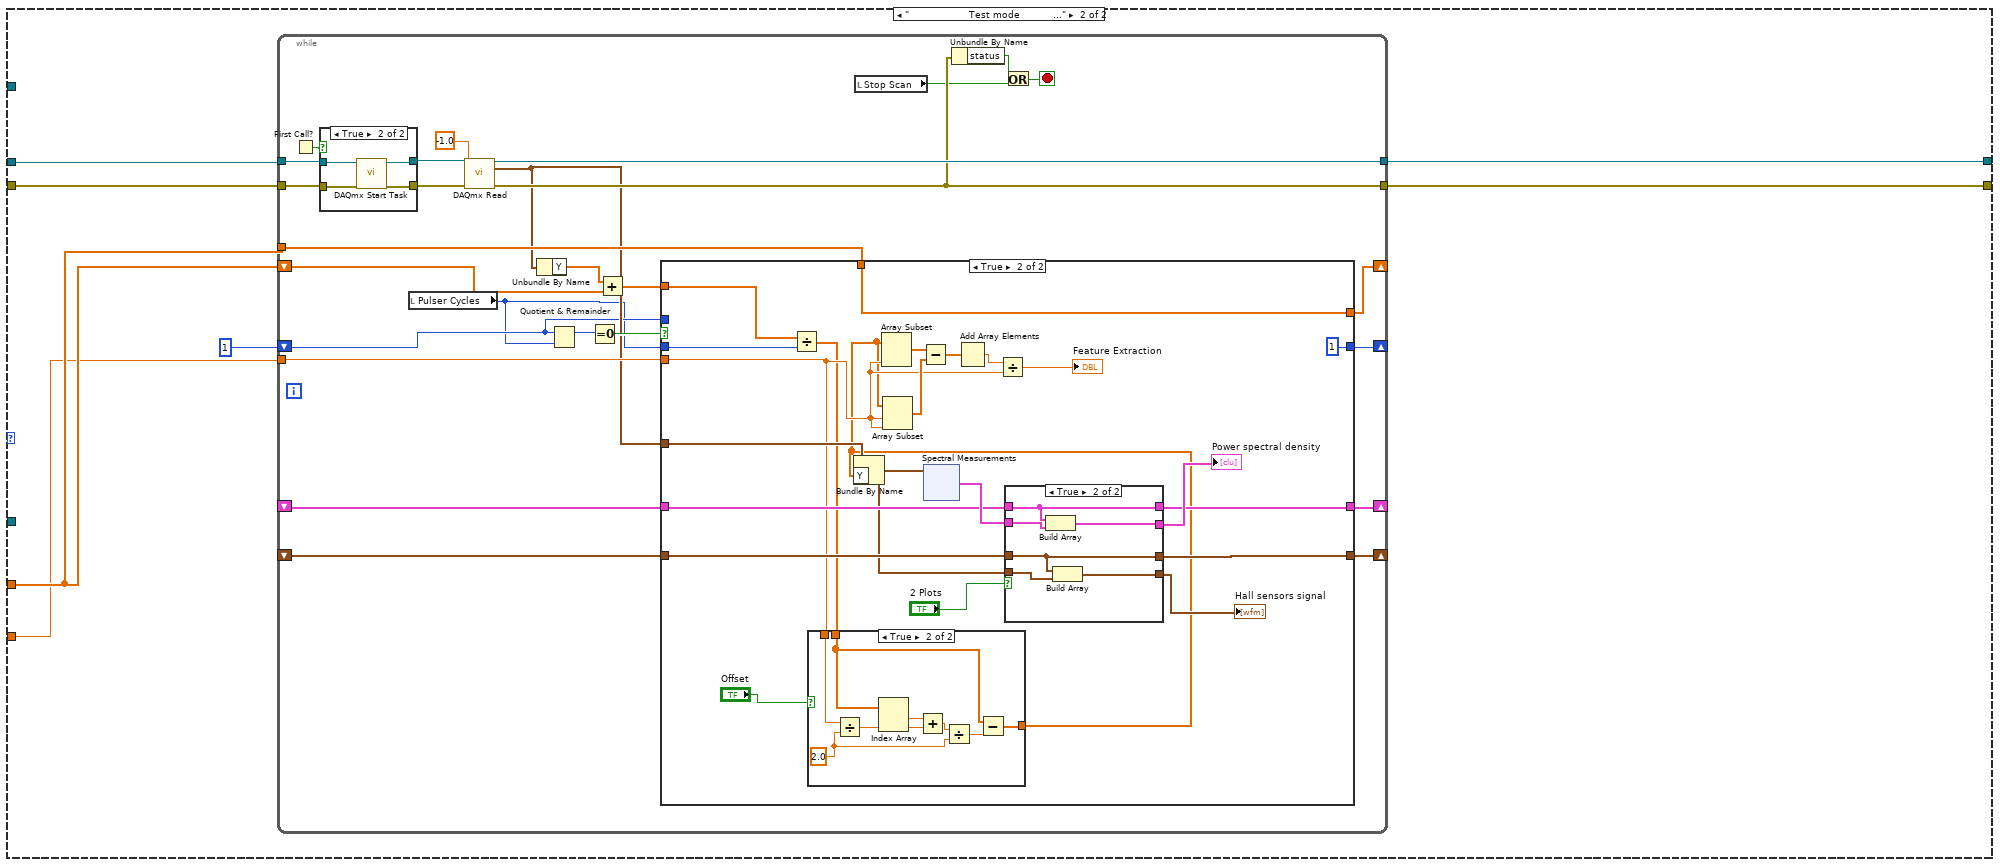
[diagram p13: hidden frame]
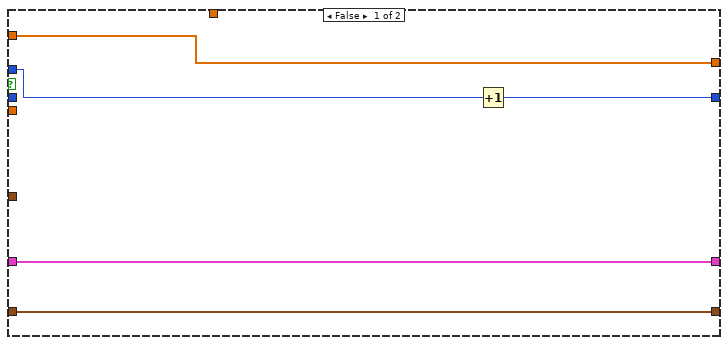
[diagram p15: hidden frame]
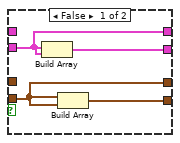
[diagram p17: hidden frame]
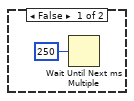
[diagram p18: hidden frame]
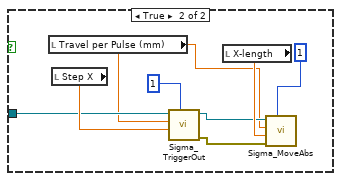
[diagram p19: hidden frame]
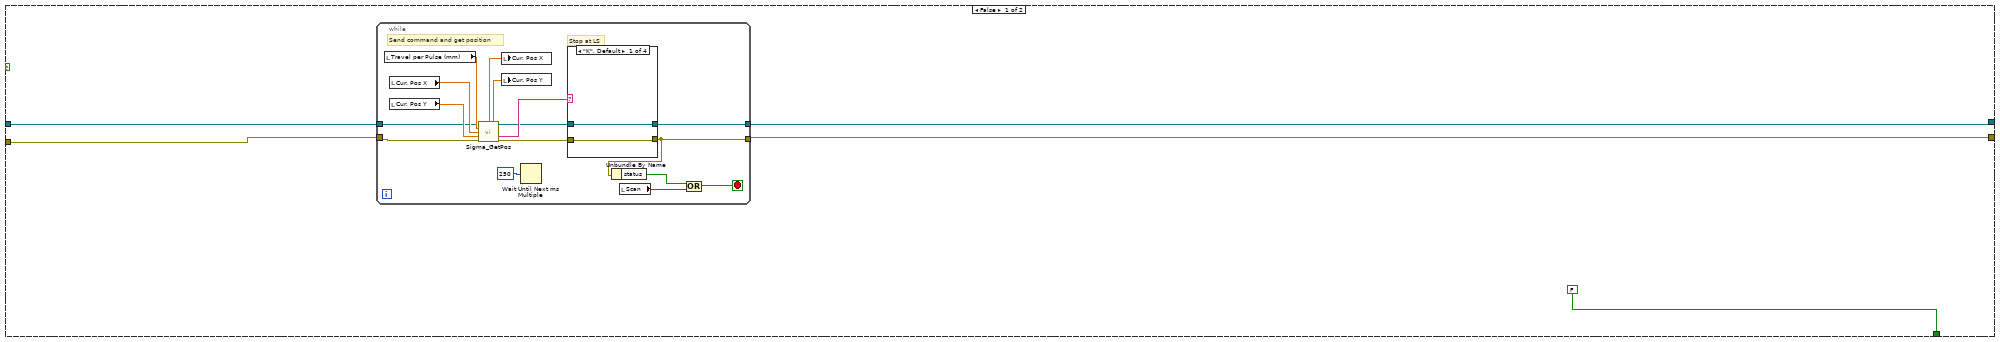
[diagram p20: hidden frame]
diagram:
  w28 = 10280 items=["상승"=10280, "하강"=10171] ("edge")
  w43 = 10178 items=["Finite Samples"=10178, "Continuous Samples"=10123, "Hardware Timed Single Point"=12522]  # Sample Mode
  w72 = 10178 items=["Finite Samples"=10178, "Continuous Samples"=10123, "Hardware Timed Single Point"=12522]  # Sample Mode
  w87 = 15846 items=["Open"=10437, "Open or Create"=15846, "Create or Replace"=15847, "Create"=15848]  # Operation
  # "No. step = 5\n1p~0.004mm"
  # "Initial speed for 2 axes"
  # "Sigma Control"
  n1 = local read "Output Array"() -> (w12:T3)
  n2 = call-poly <vilib>:"DAQmx Create Virtual Channel.vi"("maximum value"="Max Voltage", "minimum value"="Min Voltage", "input terminal configuration"="Terminal Configuration", "physical channels"="Physical Channel") -> ("task out"=w90:refnum<k21>, "error out"=w91:errorcluster)  [unwired: 10 in]
  n3 = Index Array(array=w12) -> (element=w9:T4)  [unwired: 1 in]
  n4 = Unbundle By Name(w9) -> ("Frequency"=w10:dbl)
  n5 = Divide(x="Sample Rate", y=w10) -> (x/y=w6:dbl)
  n6 = Round Toward -Infinity(1:w6) -> (0:w5:dbl)
  "Sample per Channel AI" <- w5
  n7 = call-poly <vilib>:"DAQmx Timing.vi"("task/channels in"=w90, "sample mode"=w72, "samples per channel"=w5, "rate"="Sample Rate", "source"="Sample Clock Source 2", "error in"=w91) -> ("task out"=w93:refnum<k21>, "error out"=w92:errorcluster)  [unwired: 8 in]
  n8 = property class="DAQmx Timing"(reference=w93, error in=w92) -> (reference out=w89:refnum<k21>, error out=w88:errorcluster, "SampClk.Rate"=→"Actual Sample Rate":dbl)
  n9 = local read "Output Array"() -> (w67:T3)
  n10 = call-poly <vilib>:"DAQmx Configure Logging.vi"("task/channels in"=w89, "operation"=w87, "file path"="TDMS File Path", "logging mode"="Logging Mode", "error in"=w88) -> ("task out"=w86:refnum<k21>, "error out"=w85:errorcluster)  [unwired: 9 in]
  n11 = Index Array(array=w67) -> (element=w66:T4)  [unwired: 1 in]
  n12 = disable-structure shown="비활성화" {
    frame Disabled {
      n13 = local read "Step X"() -> (w118:dbl)
      n14 = Add(x="X-length count", y=w118) -> (x+y=w117:dbl)
      n15 = local write "X-length"(w117) -> ()
    }
    frame Enabled {
    }
  }
  n16 = Unbundle By Name(w66) -> ("Frequency"=w65:dbl)
  n17 = local read "Output Array"() -> (w16:T3)
  n18 = call-poly <vilib>:"DAQmx Trigger.vi"("task/channels in"=w86, "source"="Digital Trigger Source", "edge"="Edge", "error in"=w85) -> ("task out"=w69:refnum<k21>, "error out"=w68:errorcluster)  [unwired: 10 in]
  n19 = call-poly "VISA Configure Serial Port"("VISA resource name"="COM Port", "baud rate (9600)"="Baud Rate", "data bits (8)"="Data bits", "parity (0:none)"="Parity", "stop bits (10: 1 bit)"="stop bits") -> ("VISA resource name out"=w102:refnum<visa-resource-name>, "error out"=w96:errorcluster)  [unwired: 9 in]
  n20 = Divide(x="Sample Rate", y=w65) -> (x/y=w64:dbl)
  n21 = property class="DAQmx Trigger"(reference=w69, error in=w68, "Start.Retriggerable"=TRUE) -> (reference out=w2:refnum<k21>, error out=w1:errorcluster)
  n22 = Index Array(array=w16) -> (element=w17:T4)  [unwired: 1 in]
  n23 = local read "Y-length"() -> (w50:dbl)
  n24 = local read "Step Y"() -> (w51:dbl)
  n25 = local read "X-length"() -> (w53:dbl)
  n26 = local read "Step X"() -> (w52:dbl)
  n27 = Divide(x=w64, y=2.0) -> (x/y=w62:dbl)
  n28 = call-poly <vilib>:"DAQmx Create Virtual Channel.vi"("maximum value"="Max Voltage 2", "minimum value"="Min Voltage 2", "physical channels"="Physical Channel(s)", "error in"=w1) -> ("task out"=w27:refnum<k21>, "error out"=w26:errorcluster)  [unwired: 10 in]
  n29 = Unbundle By Name(w17) -> ("Frequency"=w18:dbl)
  n30 = VISA Set I/O Buffer Size(VISA resource name=w102, mask (16)=48, size (4096)=u32 8192, error in (no error)=w96) -> (VISA resource name out=w106:refnum<visa-resource-name>, error out=w105:errorcluster)
  n31 = Quotient & Remainder(x=w50, y=w51) -> (floor(x/y)=w49:dbl)  [unwired: 1 out]
  n32 = Quotient & Remainder(x=w53, y=w52) -> (floor(x/y)=w3:dbl)  [unwired: 1 out]
  n33 = Obtain Queue(max queue size (-1, unlimited)=10000, name (unnamed)="data DAQ", element data type=dbl[] [] ("data")) -> (queue out=w58:refnum<queue>)  [unwired: 2 in, 2 out]
  n34 = Increment(x=w49) -> (x+1=w4:dbl)
  n35 = Divide(x="Sample Rate 2", y=w18) -> (x/y=w14:dbl)
  n36 = Initialize Array(0.0 ("element"), w5) -> (w59:dbl[])
  n37 = Obtain Queue(max queue size (-1, unlimited)=10000, name (unnamed)="data Extraction", element data type=0.0) -> (queue out=w56:refnum<queue>)  [unwired: 2 in, 2 out]
  n38 = Multiply(x="Pulser Cycles", y=w14) -> (x*y=w8:dbl)
  n39 = Round Toward -Infinity(1:w8) -> (0:w7:dbl)
  "Sample per Channel AO" <- w7
  n40 = call-poly <vilib>:"DAQmx Timing.vi"("task/channels in"=w27, "sample mode"=w43, "samples per channel"=w7, "rate"="Sample Rate 2", "source"="Sample Clock Source", "error in"=w26) -> ("task out"=w45:refnum<k21>, "error out"=w44:errorcluster)  [unwired: 8 in]
  n41 = case shown="\"                          Scan mode                      \", Default" "Tab Control 2" {
    tunnel: w2 -> [w141 w280]
    tunnel: [w140 w279] -> w75
    tunnel: [w139 w278] -> w74
    tunnel: w59 -> [w136 w277]
    tunnel: w1 -> [w138 w276]
    tunnel: w62 -> [w137 w275]
    tunnel: w58 -> [w135 _]
    tunnel: w56 -> [w126 _]
    tunnel: w3 -> [w133 _]
    tunnel: w4 -> [w132 _]
    frame "                          Scan mode                      ", Default {
      # "Column"
      # "Row"
      n42 = local read "3D Surface"() -> (w119:refnum<k7>)
      n43 = Initialize Array(0.0 ("element"), w133, w132) -> (w125:dbl[][])
      n44 = Matrix Size(0:w125) -> (1:w127:i32, 2:w128:i32)
      n45 = Decrement(x=w127) -> (x-1=w131:i32)
      n46 = Decrement(x=w128) -> (x-1=w130:i32)
      n47 = call "Surface_AxesScale.vi"("Y-axis Max"=w130, "X-axis max"=w131, "3D Surface"=w119, "Auto Scale"=FALSE) -> ()  [unwired: 8 in]
      n48 = while {
        shift-right: [w162] -> _
        shift-left: 0 -> [w164]
        shift-right: [w161] -> _
        shift-left: 0 -> [w163]
        tunnel: w126 -> [w160]
        shift-right: [w152] -> w120
        shift-left: w125 -> [w159]
        shift-right: [w153] -> _
        shift-left: TRUE ("Output Direction") -> [w154]
        stop <- w156 stop-if-true
        n49 = local read "Scan"() -> (w158:bool)
        n50 = case shown="True" w158 {
          tunnel: w164 -> [w172 w190]
          tunnel: w163 -> [w171 w189]
          tunnel: [w172 w188] -> w162
          tunnel: [w171 w187] -> w161
          tunnel: w160 -> [_ w186]
          tunnel: w159 -> [w166 w184]
          tunnel: [w167 w180] -> w152
          tunnel: [_ w183] -> w155
          tunnel: w154 -> [w170 w182]
          tunnel: [w170 w181] -> w153
          frame False {
            n51 = call "CSV Open.vi"("Open"="Open") -> ("2D Array Out"=w169:dbl[][])  [unwired: 10 in]
            n52 = case shown="True" "Open" {
              tunnel: w169 -> [_ w174]
              tunnel: [w173 w174] -> w167
              tunnel: w166 -> [w173 _]
              frame False {
              }
              frame True {
                n53 = Matrix Size(0:w174) -> (1:w175:i32, 2:w176:i32)
                n54 = Decrement(x=w175) -> (x-1=w179:i32)
                n55 = Decrement(x=w176) -> (x-1=w178:i32)
                n56 = call "Surface_AxesScale.vi"("Y-axis Max"=w178, "X-axis max"=w179, "Auto Scale"=FALSE) -> ()  [unwired: 9 in]
              }
            }
            n57 = Wait Until Next ms Multiple(millisecond multiple=u32 100 ("ms 배수")) -> ()  [unwired: 1 out]
          }
          frame True {
            n58 = Dequeue Element(queue=w186) -> (element=w185:dbl)  [unwired: 2 in, 3 out]
            n59 = call "EletoMatr_1channel.vi"("Input Array X"=w184, "Input data"=w185, "In Row"=w190, "In Column"=w189, "Input Direction"=w182) -> ("Completed"=w183:bool, "Out Array X"=w180:dbl[][], "Out Row"=w188:i32, "Output Direction"=w181:bool, "Out Column"=w187:i32)  [unwired: 6 in]
          }
        }
        n60 = local read "Stop Scan"() -> (w157:bool)
        n61 = global write "Global_data.vi" "global 2d graph"(w152) -> ()
        n62 = Compound Arithmetic op=OR(w155, w157) -> (w156:bool)
      }
      n63 = while {
        tunnel: w141 -> [w197]
        tunnel: [w196] -> w140
        tunnel: [w195] -> w139
        tunnel: w138 -> [w194]
        tunnel: w135 -> [w193]
        stop <- w192 stop-if-true
        n64 = case shown="True" "Scan" {
          tunnel: w197 -> [w199 w204]
          tunnel: [w199 w203] -> w196
          tunnel: [w198 w202] -> w195
          tunnel: w194 -> [w198 w201]
          tunnel: w193 -> [_ w200]
          frame False {
          }
          frame True {
            n65 = while {
              tunnel: w204 -> [w209]
              tunnel: [w216] -> w203
              tunnel: [w215] -> w202
              tunnel: w201 -> [w208]
              tunnel: w200 -> [w214]
              tunnel: [w210] -> _
              stop <- w212 stop-if-true
              n66 = First Call?() -> (First Call?: T/F=w205:bool)
              n67 = case shown="True" w205 {
                tunnel: w209 -> [w217 w222]
                tunnel: w208 -> [w218 w221]
                tunnel: [w217 w220] -> w207
                tunnel: [w218 w219] -> w206
                frame False {
                }
                frame True {
                  n68 = call <vilib>:"DAQmx Start Task.vi"("task/channels in"=w222, "error in"=w221) -> ("task out"=w220:refnum<k21>, "error out"=w219:errorcluster)  [unwired: 12 in]
                }
              }
              n69 = call-poly <vilib>:"DAQmx Read.vi"("task/channels in"=w207, "error in"=w206) -> ("task out"=w216:refnum<k21>, "data"=w211:dbl[], "error out"=w215:errorcluster)  [unwired: 11 in]
              n70 = Enqueue Element(queue=w214, element=w211) -> ()  [unwired: 2 in, 3 out]
              n71 = local read "Stop Scan"() -> (w210:bool)
              n72 = Unbundle By Name(w215) -> ("status"=w213:bool)
              n73 = Or(x=w213, y=w210) -> (x .or. y?=w212:bool)
            }
          }
        }
        n74 = local read "Stop Scan"() -> (w192:bool)
      }
      n75 = while {
        shift-right: [w228] -> _
        shift-left: w136 -> [w232]
        tunnel: w136 -> [w231]
        tunnel: w137 -> [w230]
        tunnel: w135 -> [w229]
        tunnel: w126 -> [w227]
        shift-right: [w224] -> _
        shift-left: 0 -> [w225]
        stop <- w223 stop-if-true
        n76 = local read "Scan"() -> (w226:bool)
        n77 = case shown="True" w226 {
          tunnel: w232 -> [w235 w239]
          tunnel: w231 -> [_ w245]
          tunnel: w230 -> [_ w244]
          tunnel: w229 -> [_ w243]
          tunnel: [w235 w242] -> w228
          tunnel: w227 -> [_ w241]
          tunnel: w225 -> [w234 w237]
          tunnel: [w234 w236] -> w224
          frame False {
            n78 = Wait Until Next ms Multiple(millisecond multiple=u32 100 ("ms 배수")) -> ()  [unwired: 1 out]
          }
          frame True {
            n79 = local read "Pulser Cycles"() -> (w238:i32)
            n80 = Increment(x=w237) -> (x+1=w236:i32)
            n81 = Dequeue Element(queue=w243) -> (element=w240:dbl[])  [unwired: 2 in, 3 out]
            n82 = Quotient & Remainder(x=w236, y=w238) -> (x-y*floor(x/y)=w246:i32)  [unwired: 1 out]
            n83 = Add(x=w240, y=w239) -> (x+y=w248:dbl[])
            n84 = Equal To 0?(x=w246) -> (x = 0?=w247:bool)
            n85 = case shown="False" w247 {
              tunnel: w238 -> [_ w257]
              tunnel: w248 -> [w249 w263]
              tunnel: [w249 w262] -> w242
              tunnel: w245 -> [_ w262]
              tunnel: w244 -> [_ w256]
              tunnel: w241 -> [_ w254]
              frame False {
                n86 = disable-structure shown="비활성화" {
                  frame Disabled {
                    n87 = Wait Until Next ms Multiple(millisecond multiple=u32 100 ("ms 배수")) -> ()  [unwired: 1 out]
                  }
                  frame Enabled {
                  }
                }
              }
              frame True {
                n88 = local read "Offset"() -> (w252:bool)
                n89 = Divide(x=w263, y=w257) -> (x/y=w253:dbl[])
                n90 = case shown="True" w252 {
                  tunnel: w256 -> [_ w272]
                  tunnel: w253 -> [w264 w266]
                  tunnel: [w264 w265] -> w255
                  frame False {
                  }
                  frame True {
                    w268 = 2.0 ("y")
                    n91 = Divide(x=w272, y=w268) -> (x/y=w273:dbl)
                    n92 = Index Array(array=w266, index #2=w273) -> (element #1=w270:dbl, element #2=w271:dbl)  [unwired: 1 in]
                    n93 = Add(x=w270, y=w271) -> (x+y=w269:dbl)
                    n94 = Divide(x=w269, y=w268) -> (x/y=w267:dbl)
                    n95 = Subtract(x=w266, y=w267) -> (x-y=w265:dbl[])
                  }
                }
                n96 = Array Subset(array=w255, length=w256) -> (w260:dbl[])  [unwired: 1 in]
                n97 = Array Subset(array=w255, index=w256, length=w256) -> (w259:dbl[])
                n98 = Subtract(x=w260, y=w259) -> (x-y=w258:dbl[])
                n99 = Add Array Elements(numeric array=w258) -> (sum=w261:dbl)
                n100 = Divide(x=w261, y=w256) -> (x/y=w251:dbl)
                "Feature Extraction 2" <- w251
                n101 = Enqueue Element(queue=w254, element=w251) -> ()  [unwired: 2 in, 3 out]
              }
            }
          }
        }
        n102 = local read "Stop Scan"() -> (w223:bool)
        "No.data" <- w225
      }
      n103 = while {
        stop <- w146 stop-if-true
        n104 = global read "Global_data.vi" "global 2d graph"() -> (w142:dbl[][])
        n105 = Wait (ms)(milliseconds to wait=u32 100) -> ()  [unwired: 1 out]
        n106 = call <vilib>:"3D Surface.vi"("z matrix"=w142, "3D graph"="3D Surface") -> ()  [unwired: 8 in, 2 out]
        n107 = local read "3D Surface"() -> (w148:refnum<k7>)
        n108 = property class="CWGraph3D"(reference=w148, "ViewMode"="ViewMode") -> ()  [unwired: 1 in, 2 out]
        n109 = call <vilib>:"Basic Properties.vi"("3D graph"=w148, "plot style"="Plot style") -> ()  [unwired: 12 in, 2 out]
        n110 = local read "Stop Scan"() -> (w146:bool)
      }
      n111 = while {
        tunnel: w120 -> [w150]
        stop <- w149 stop-if-true
        n112 = call "CSV Save.vi"("Array"=w150, "Save Button"="Save Scan mode") -> ("Save Status"=w149:bool)  [unwired: 9 in]
      }
    }
    frame "                    Test mode                   " {
      n113 = while {
        tunnel: w280 -> [w284]
        tunnel: w276 -> [w283]
        tunnel: [w305] -> w278
        tunnel: [w306] -> w279
        shift-right: [w300] -> _
        shift-left: w277 -> [w301]
        tunnel: w277 -> [w299]
        shift-right: [w297] -> _
        shift-left: _ -> [w296]
        tunnel: w275 -> [w295]
        shift-right: [w294] -> _
        shift-left: _ -> [w293]
        shift-right: [w288] -> _
        shift-left: 1 ("Average") -> [w287]
        stop <- w307 stop-if-true
        n114 = First Call?() -> (First Call?: T/F=w285:bool)
        n115 = case shown="True" w285 {
          tunnel: w284 -> [w308 w313]
          tunnel: w283 -> [w309 w312]
          tunnel: [w308 w311] -> w282
          tunnel: [w309 w310] -> w281
          frame False {
          }
          frame True {
            n116 = call <vilib>:"DAQmx Start Task.vi"("task/channels in"=w313, "error in"=w312) -> ("task out"=w311:refnum<k21>, "error out"=w310:errorcluster)  [unwired: 12 in]
          }
        }
        n117 = local read "Pulser Cycles"() -> (w286:i32)
        n118 = call-poly <vilib>:"DAQmx Read.vi"("task/channels in"=w282, "timeout"=-1.0, "error in"=w281) -> ("task out"=w306:refnum<k21>, "data"=w289:waveform(dbl), "error out"=w305:errorcluster)  [unwired: 10 in]
        n119 = Unbundle By Name(w289) -> ("Y"=w292:dbl[])
        n120 = Quotient & Remainder(x=w287, y=w286) -> (x-y*floor(x/y)=w303:i32)  [unwired: 1 out]
        n121 = Equal To 0?(x=w303) -> (x = 0?=w302:bool)
        n122 = Add(x=w292, y=w301) -> (x+y=w298:dbl[])
        n123 = case shown="True" w302 {
          tunnel: w286 -> [_ w320]
          tunnel: w289 -> [_ w341]
          tunnel: w298 -> [w318 w340]
          tunnel: [w318 w339] -> w300
          tunnel: w299 -> [_ w339]
          tunnel: [w317 w335] -> w297
          tunnel: w296 -> [w317 w337]
          tunnel: w295 -> [_ w324]
          tunnel: [w316 w330] -> w294
          tunnel: w293 -> [w316 w332]
          tunnel: [w314 1 ("Average")] -> w288
          tunnel: w287 -> [w315 _]
          frame False {
            n124 = Increment(x=w315) -> (x+1=w314:i32)
          }
          frame True {
            n125 = Divide(x=w340, y=w320) -> (x/y=w323:dbl[])
            n126 = case shown="True" "Offset" {
              tunnel: w324 -> [_ w350]
              tunnel: w323 -> [w342 w344]
              tunnel: [w342 w343] -> w321
              frame False {
              }
              frame True {
                w346 = 2.0 ("y")
                n127 = Divide(x=w350, y=w346) -> (x/y=w351:dbl)
                n128 = Index Array(array=w344, index #2=w351) -> (element #1=w348:dbl, element #2=w349:dbl)  [unwired: 1 in]
                n129 = Add(x=w348, y=w349) -> (x+y=w347:dbl)
                n130 = Divide(x=w347, y=w346) -> (x/y=w345:dbl)
                n131 = Subtract(x=w344, y=w345) -> (x-y=w343:dbl[])
              }
            }
            n132 = Bundle By Name(cluster=w341, "Y"=w321) -> (w329:waveform(dbl))
            n133 = Array Subset(array=w321, length=w324) -> (w328:dbl[])  [unwired: 1 in]
            n134 = Array Subset(array=w321, index=w324, length=w324) -> (w327:dbl[])
            n135 = Subtract(x=w328, y=w327) -> (x-y=w326:dbl[])
            n136 = xnode "Spectral Measurements"("신호"=w329) -> ("PSD"=w333:cluster{"f0":dbl, "df":dbl, "magnitude":dbl[]})  [unwired: 1 in, 1 out]
            n137 = Add Array Elements(numeric array=w326) -> (sum=w334:dbl)
            n138 = Divide(x=w334, y=w324) -> (x/y=→"Feature Extraction":dbl)
            n139 = case shown="True" "2 Plots" {
              tunnel: [w355 w361] -> w338
              tunnel: w337 -> [_ w360]
              tunnel: [w354 w360] -> w335
              tunnel: w329 -> [w354 w356]
              tunnel: w333 -> [w352 w358]
              tunnel: [w353 w359] -> w331
              tunnel: w332 -> [_ w357]
              tunnel: [w352 w357] -> w330
              frame False {
                n140 = Build Array(w352, w352) -> (w353:cluster{"f0":dbl, "df":dbl, "magnitude":dbl[]}[])
                n141 = Build Array(w354, w354) -> (w355:waveform(dbl)[])
              }
              frame True {
                n142 = Build Array(w357, w358) -> (w359:cluster{"f0":dbl, "df":dbl, "magnitude":dbl[]}[])
                n143 = Build Array(w360, w356) -> (w361:waveform(dbl)[])
              }
            }
            "Power spectral density" <- w331
            "Hall sensors signal" <- w338
          }
        }
        n144 = local read "Stop Scan"() -> (w291:bool)
        n145 = Unbundle By Name(w305) -> ("status"=w304:bool)
        n146 = Or(x=w304, y=w291) -> (x .or. y?=w307:bool)
      }
    }
  }
  n147 = property class="DAQmx Timing"(reference=w45, error in=w44) -> (reference out=w31:refnum<k21>, error out=w37:errorcluster, "SampClk.Rate"=w35:dbl)
  "Actual Sample Rate 2" <- w35
  n148 = call "Sigma_SetSpeed.vi"("VISA resource name"=w106, "Travel per Pulse (0.004mm)"="Travel per Pulse (mm)", "Min (1mm) 2"="2 Min", "Max (2mm) 2"="2 Max", "Rate (1mm) 2"="2 Rate", "error in (no error)"=w105, "Axis (1)"="W", "Min (1mm)"="1 Min", "Max (2mm)"="1  Max", "Rate (1mm)"="1 Rate") -> ("VISA resource name out"=w94:refnum<visa-resource-name>, "error out"=w95:errorcluster)  [unwired: 8 in]
  n149 = Bundle By Name(cluster=cluster{"Fs":dbl, "#s":dbl} {"Fs"=1000.0, "#s"=1000.0} ("sampling info"), "#s"=w7, "Fs"=w35) -> (w34:cluster{"Fs":dbl, "#s":dbl})
  n150 = for {
    tunnel: w37 -> [w379]
    tunnel: w34 -> [w378]
    tunnel: [w377] -> w30
    tunnel: "Output Array" -> [w376] mode=indexing
    tunnel: [w373] -> w33 mode=indexing
    n151 = Unbundle By Name(w376) -> ("Waveform Type"=w375:u16, "Frequency"=w374:dbl, "Amplitude"=w371:dbl)
    n152 = call <vilib>:"Basic Function Generator.vi"("square wave duty cycle (%)"="Duty cycle %", "sampling info"=w378, "signal type"=w375, "error in (no error)"=w379, "amplitude"=w371, "frequency"=w374) -> ("error out"=w377:errorcluster, "signal out"=w373:waveform(dbl))  [unwired: 3 in, 1 out]
  }
  "Waveform Graph 2" <- w33
  n153 = call-poly <vilib>:"DAQmx Trigger.vi"("task/channels in"=w31, "source"="Pulser Trigger Source", "edge"=w28, "error in"=w30) -> ("task out"=w23:refnum<k21>, "error out"=w19:errorcluster)  [unwired: 10 in]
  n154 = property class="DAQmx Trigger"(reference=w23, error in=w19, "Start.Retriggerable"=TRUE) -> (reference out=w22:refnum<k21>, error out=w21:errorcluster)
  n155 = disable-structure shown="활성화" {
    disable-tunnel: w33 -> [w384 w407]
    disable-tunnel: [w383 w406] -> w25
    disable-tunnel: [w382 w405] -> w24
    disable-tunnel: w22 -> [w381 w409]
    disable-tunnel: w21 -> [w380 w408]
    frame Disabled {
      n156 = while {
        tunnel: w384 -> [w395]
        shift-right: [w391] -> w383
        shift-left: w381 -> [w389]
        shift-right: [w390] -> w382
        shift-left: w380 -> [w388]
        stop <- FALSE stop-if-true
        n157 = call-poly <vilib>:"DAQmx Write.vi"("task/channels in"=w389, "data"=w395, "timeout"=-1.0, "error in"=w388) -> ("task out"=w394:refnum<k21>, "error out"=w393:errorcluster)  [unwired: 9 in, 1 out]
        n158 = call <vilib>:"DAQmx Start Task.vi"("task/channels in"=w394, "error in"=w393) -> ("task out"=w387:refnum<k21>, "error out"=w386:errorcluster)  [unwired: 12 in]
        n159 = disable-structure shown="활성화" {
          disable-tunnel: [w401 w403] -> w391
          disable-tunnel: [w400 w402] -> w390
          disable-tunnel: w387 -> [w399 w403]
          disable-tunnel: w386 -> [w398 w402]
          frame Disabled {
            n160 = call <vilib>:"DAQmx Wait Until Done.vi"("task/channels in"=w399, "error in"=w398) -> ("task out"=w397:refnum<k21>, "error out"=w396:errorcluster)  [unwired: 12 in]
            n161 = call <vilib>:"DAQmx Stop Task.vi"("task/channels in"=w397, "error in"=w396) -> ("task out"=w401:refnum<k21>, "error out"=w400:errorcluster)  [unwired: 12 in]
          }
          frame Enabled {
          }
        }
      }
    }
    frame Enabled {
      n162 = call-poly <vilib>:"DAQmx Write.vi"("task/channels in"=w409, "data"=w407, "timeout"=-1.0, "error in"=w408) -> ("task out"=w411:refnum<k21>, "error out"=w413:errorcluster)  [unwired: 9 in, 1 out]
      n163 = call <vilib>:"DAQmx Start Task.vi"("task/channels in"=w411, "error in"=w413) -> ("task out"=w410:refnum<k21>, "error out"=w412:errorcluster)  [unwired: 12 in]
      n164 = while {
        tunnel: w410 -> [w421]
        tunnel: w412 -> [w420]
        tunnel: [w418] -> w405
        tunnel: [w419] -> w406
        stop <- w414 stop-if-true
        n165 = call <vilib>:"DAQmx Is Task Done.vi"("task/channels in"=w421, "error in"=w420) -> ("task out"=w419:refnum<k21>, "error out"=w418:errorcluster)  [unwired: 11 in, 1 out]
        n166 = Unbundle By Name(w418) -> ("status"=w415:bool)
        n167 = Wait Until Next ms Multiple(millisecond multiple=u32 100) -> ()  [unwired: 1 out]
        n168 = Compound Arithmetic op=OR(w415, "Stop 4") -> (w414:bool)
      }
    }
  }
  n169 = while {
    tunnel: w94 -> [w428]
    tunnel: [w423] -> _
    tunnel: w95 -> [w427]
    tunnel: [w425] -> w115
    stop <- w424 stop-if-true
    n170 = event shown="[9] \"Emergency Stop\": Value Change" {
      selector: _ -> [_ _ _ _ _ _ _ _ _ _]
      dyn-events: _ -> [_ _ _ _ _ _ _ _ _ _]
      timeout: _ -> [_ _ _ _ _ _ _ _ _ _]
      tunnel: w428 -> [w430 w443 w446 w461 w476 w491 w508 w520 w530 w542]
      tunnel: w427 -> [w429 w440 w445 w460 w475 w490 w507 w519 w529 w541]
      tunnel: [w430 w442 w448 w463 w478 w493 w505 w518 w532 w544] -> w423
      tunnel: [w429 w441 w447 w462 w477 w492 w504 w517 w531 w543] -> w425
      tunnel: ["Stop Scan" _ _ _ _ _ _ _ _ _] -> w422
      event "Stop Scan": Value Change {
        n171 = event-data() -> ()  [unwired: 1 in, 2 out]
      }
      event "Save Speed": Value Change {
        n172 = event-data() -> ()  [unwired: 1 in, 5 out]
        n173 = local read "Travel per Pulse (mm)"() -> (w432:dbl)
        n174 = local read "1  Max"() -> (w437:dbl)
        n175 = local read "1 Rate"() -> (w436:dbl)
        n176 = local read "2 Rate"() -> (w433:dbl)
        n177 = local read "2 Max"() -> (w434:dbl)
        n178 = local read "1 Min"() -> (w438:dbl)
        n179 = local read "2 Min"() -> (w435:dbl)
        n180 = call "Sigma_SetSpeed.vi"("VISA resource name"=w443, "Travel per Pulse (0.004mm)"=w432, "Min (1mm) 2"=w435, "Max (2mm) 2"=w434, "Rate (1mm) 2"=w433, "error in (no error)"=w440, "Axis (1)"="W", "Min (1mm)"=w438, "Max (2mm)"=w437, "Rate (1mm)"=w436) -> ("VISA resource name out"=w442:refnum<visa-resource-name>, "error out"=w441:errorcluster)  [unwired: 8 in]
      }
      event "Right": Value Change {
        n181 = event-data() -> ()  [unwired: 1 in, 1 out]
        n182 = case shown="True" "Right" {
          tunnel: [w450 w456] -> w448
          tunnel: [w449 w455] -> w447
          tunnel: w446 -> [w450 w458]
          tunnel: w445 -> [w449 w457]
          frame False {
          }
          frame True {
            n183 = local read "Travel per Pulse (mm)"() -> (w452:dbl)
            n184 = local read "Move Distance (mm)"() -> (w451:dbl)
            n185 = call "Sigma_MoveAbs.vi"("Direction (+)"=FALSE, "Axis (1)"=1, "error in (no error)"=w457, "Travel (1mm)"=w451, "Travel per Pulse (0.004mm)"=w452, "VISA resource name"=w458) -> ("error out"=w455:errorcluster, "VISA resource name out"=w456:refnum<visa-resource-name>)  [unwired: 4 in]
          }
        }
      }
      event "Left": Value Change {
        n186 = event-data() -> ()  [unwired: 1 in, 1 out]
        n187 = case shown="True" "Left" {
          tunnel: [w465 w472] -> w463
          tunnel: [w464 w471] -> w462
          tunnel: w461 -> [w465 w473]
          tunnel: w460 -> [w464 w470]
          frame False {
          }
          frame True {
            n188 = local read "Travel per Pulse (mm)"() -> (w467:dbl)
            n189 = local read "Move Distance (mm)"() -> (w466:dbl)
            n190 = call "Sigma_MoveAbs.vi"("Direction (+)"=TRUE, "Axis (1)"=1, "error in (no error)"=w470, "Travel (1mm)"=w466, "Travel per Pulse (0.004mm)"=w467, "VISA resource name"=w473) -> ("error out"=w471:errorcluster, "VISA resource name out"=w472:refnum<visa-resource-name>)  [unwired: 4 in]
          }
        }
      }
      event "Front": Value Change {
        n191 = event-data() -> ()  [unwired: 1 in, 1 out]
        n192 = case shown="True" "Front" {
          tunnel: [w480 w486] -> w478
          tunnel: [w479 w485] -> w477
          tunnel: w476 -> [w480 w488]
          tunnel: w475 -> [w479 w487]
          frame False {
          }
          frame True {
            n193 = local read "Travel per Pulse (mm)"() -> (w482:dbl)
            n194 = local read "Move Distance (mm)"() -> (w481:dbl)
            n195 = call "Sigma_MoveAbs.vi"("Direction (+)"=FALSE, "Axis (1)"=2, "error in (no error)"=w487, "Travel (1mm)"=w481, "Travel per Pulse (0.004mm)"=w482, "VISA resource name"=w488) -> ("error out"=w485:errorcluster, "VISA resource name out"=w486:refnum<visa-resource-name>)  [unwired: 4 in]
          }
        }
      }
      event "Back": Value Change {
        n196 = event-data() -> ()  [unwired: 1 in, 1 out]
        n197 = case shown="True" "Back" {
          tunnel: [w495 w501] -> w493
          tunnel: [w494 w500] -> w492
          tunnel: w491 -> [w495 w503]
          tunnel: w490 -> [w494 w502]
          frame False {
          }
          frame True {
            n198 = local read "Travel per Pulse (mm)"() -> (w497:dbl)
            n199 = local read "Move Distance (mm)"() -> (w496:dbl)
            n200 = call "Sigma_MoveAbs.vi"("Direction (+)"=TRUE, "Axis (1)"=2, "error in (no error)"=w502, "Travel (1mm)"=w496, "Travel per Pulse (0.004mm)"=w497, "VISA resource name"=w503) -> ("error out"=w500:errorcluster, "VISA resource name out"=w501:refnum<visa-resource-name>)  [unwired: 4 in]
          }
        }
      }
      event "Home X": Value Change {
        n201 = event-data() -> ()  [unwired: 1 in, 1 out]
        n202 = case shown="True" "Home X" {
          tunnel: [w510 w513] -> w505
          tunnel: [w509 w512] -> w504
          tunnel: w508 -> [w510 w515]
          tunnel: w507 -> [w509 w514]
          frame False {
          }
          frame True {
            n203 = call "Sigma_Home.vi"("Axis (1)"="1", "error in (no error)"=w514, "VISA resource name"=w515) -> ("error out"=w512:errorcluster, "VISA resource name out"=w513:refnum<visa-resource-name>)  [unwired: 7 in]
          }
        }
      }
      event "Home Y": Value Change {
        n204 = event-data() -> ()  [unwired: 1 in, 1 out]
        n205 = case shown="True" "Home Y" {
          tunnel: [w522 w525] -> w518
          tunnel: [w521 w524] -> w517
          tunnel: w520 -> [w522 w527]
          tunnel: w519 -> [w521 w526]
          frame False {
          }
          frame True {
            n206 = call "Sigma_Home.vi"("Axis (1)"="2", "error in (no error)"=w526, "VISA resource name"=w527) -> ("error out"=w524:errorcluster, "VISA resource name out"=w525:refnum<visa-resource-name>)  [unwired: 7 in]
          }
        }
      }
      event "Stop 3": Value Change {
        n207 = event-data() -> ()  [unwired: 1 in, 1 out]
        n208 = case shown="True" "Stop 3" {
          tunnel: [w534 w535] -> w532
          tunnel: [w533 w536] -> w531
          tunnel: w530 -> [w534 w538]
          tunnel: w529 -> [w533 w537]
          frame False {
          }
          frame True {
            n209 = call "Sigma_Stop.vi"("Axis (1)"="W", "error in (no error)"=w537, "VISA resource name"=w538) -> ("error out"=w536:errorcluster, "VISA resource name out"=w535:refnum<visa-resource-name>)  [unwired: 7 in]
          }
        }
      }
      event "Emergency Stop": Value Change {
        n210 = event-data() -> ()  [unwired: 1 in, 1 out]
        n211 = case shown="True" "Emergency Stop" {
          tunnel: [w546 w549] -> w544
          tunnel: [w545 w548] -> w543
          tunnel: w542 -> [w546 w551]
          tunnel: w541 -> [w545 w550]
          frame False {
          }
          frame True {
            n212 = call "Sigma_Stop.vi"("Axis (1)"="E", "error in (no error)"=w550, "VISA resource name"=w551) -> ("error out"=w548:errorcluster, "VISA resource name out"=w549:refnum<visa-resource-name>)  [unwired: 7 in]
          }
        }
      }
    }
    n213 = Unbundle By Name(w425) -> ("status"=w426:bool)
    n214 = Compound Arithmetic op=OR(w426, w422) -> (w424:bool)
  }
  n215 = call <vilib>:"DAQmx Clear Task.vi"("task in"=w25, "error in"=w24) -> ("error out"=w42:errorcluster)  [unwired: 13 in]
  n216 = call <vilib>:"Simple Error Handler.vi"("error in (no error)"=w42) -> ()  [unwired: 4 in, 5 out]
  n217 = call <vilib>:"DAQmx Clear Task.vi"("task in"=w75, "error in"=w74) -> ("error out"=w84:errorcluster)  [unwired: 13 in]
  n218 = call <vilib>:"Simple Error Handler.vi"("error in (no error)"=w84) -> ()  [unwired: 4 in, 5 out]
  n219 = call <vilib>:"Simple Error Handler.vi"("error in (no error)"=w115) -> ()  [unwired: 4 in, 5 out]
  n220 = while {
    tunnel: w94 -> [w552]
    stop <- FALSE stop-if-true
    n221 = case shown="False" "Forward scan" {
      tunnel: w552 -> [_ w568]
      frame False {
        n222 = Wait Until Next ms Multiple(millisecond multiple=u32 250 ("ms 배수")) -> ()  [unwired: 1 out]
      }
      frame True {
        n223 = local read "Travel per Pulse (mm)"() -> (w567:dbl)
        n224 = local read "Step X"() -> (w573:dbl)
        n225 = call "Sigma_TriggerOut.vi"("Axis(1)"=1, "Trigger distance (mm)"=w573, "Travel per Pulse (mm)"=w567, "VISA resource name"=w568) -> ("error out"=w569:errorcluster, "VISA resource name out"=w570:refnum<visa-resource-name>)  [unwired: 6 in]
        n226 = local read "X-length"() -> (w571:dbl)
        n227 = call "Sigma_MoveAbs.vi"("Axis (1)"=1, "error in (no error)"=w569, "Travel (1mm)"=w571, "Travel per Pulse (0.004mm)"=w567, "VISA resource name"=w570) -> ()  [unwired: 5 in, 2 out]
      }
    }
    n228 = case shown="True" "Backward scan" {
      tunnel: w552 -> [_ w559]
      frame False {
        n229 = Wait Until Next ms Multiple(millisecond multiple=u32 250 ("ms 배수")) -> ()  [unwired: 1 out]
      }
      frame True {
        n230 = local read "Travel per Pulse (mm)"() -> (w558:dbl)
        n231 = local read "Step X"() -> (w564:dbl)
        n232 = call "Sigma_TriggerOut.vi"("Axis(1)"=1, "Trigger distance (mm)"=w564, "Travel per Pulse (mm)"=w558, "VISA resource name"=w559) -> ("error out"=w560:errorcluster, "VISA resource name out"=w561:refnum<visa-resource-name>)  [unwired: 6 in]
        n233 = local read "X-length"() -> (w562:dbl)
        n234 = call "Sigma_MoveAbs.vi"("Direction (+)"=FALSE, "Axis (1)"=1, "error in (no error)"=w560, "Travel (1mm)"=w562, "Travel per Pulse (0.004mm)"=w558, "VISA resource name"=w561) -> ()  [unwired: 4 in, 2 out]
      }
    }
  }
  n235 = while {
    tunnel: w94 -> [w580]
    tunnel: [w578] -> _
    tunnel: w95 -> [w579]
    tunnel: [w577] -> _
    stop <- w576 stop-if-true
    n236 = local read "Scan"() -> (w575:bool)
    n237 = case shown="True" w575 {
      selector: w575 -> [_ w626]
      tunnel: [w582 w628] -> w578
      tunnel: w580 -> [w584 w625]
      tunnel: w579 -> [w583 w622]
      tunnel: [w581 w627] -> w577
      tunnel: [FALSE w630] -> w576
      frame False {
        n238 = while {
          tunnel: w583 -> [w593]
          tunnel: [w588] -> w582
          tunnel: [w587] -> w581
          tunnel: w584 -> [w586]
          stop <- w600 stop-if-true
          # "Stop at LS"
          # "Send command and get position"
          n239 = local read "Travel per Pulse (mm)"() -> (w596:dbl)
          n240 = local read "Cur. Pos X"() -> (w590:dbl)
          n241 = local read "Cur. Pos Y"() -> (w589:dbl)
          n242 = call "Sigma_GetPos.vi"("VISA resource name"=w586, "Travel per Pulse (mm)"=w596, "Init Pos X (mm)"=w590, "Init  Pos Y (mm)"=w589, "error in (no error)"=w593) -> ("Pos X (mm)"=w592:dbl, "Pos Y (mm)"=w591:dbl, "VISA resource name out"=w595:refnum<visa-resource-name>, "State String"=w597:string, "error out"=w594:errorcluster)  [unwired: 6 in]
          n243 = local write "Cur. Pos X"(w592) -> ()
          n244 = local write "Cur. Pos Y"(w591) -> ()
          n245 = Wait Until Next ms Multiple(millisecond multiple=u32 250) -> ()  [unwired: 1 out]
          n246 = case shown="\"K\", Default" w597 {
            tunnel: [w603 w608 w613 w618] -> w588
            tunnel: [w602 w607 w612 w617] -> w587
            tunnel: w595 -> [w603 w605 w610 w615]
            tunnel: w594 -> [w602 w604 w609 w614]
            frame "K", Default {
            }
            frame "L" {
              n247 = call "Sigma_Stop.vi"("Axis (1)"="1", "error in (no error)"=w604, "VISA resource name"=w605) -> ("error out"=w607:errorcluster, "VISA resource name out"=w608:refnum<visa-resource-name>)  [unwired: 7 in]
            }
            frame "M" {
              n248 = call "Sigma_Stop.vi"("Axis (1)"="2", "error in (no error)"=w609, "VISA resource name"=w610) -> ("error out"=w612:errorcluster, "VISA resource name out"=w613:refnum<visa-resource-name>)  [unwired: 7 in]
            }
            frame "W" {
              n249 = call "Sigma_Stop.vi"("Axis (1)"="W", "error in (no error)"=w614, "VISA resource name"=w615) -> ("error out"=w617:errorcluster, "VISA resource name out"=w618:refnum<visa-resource-name>)  [unwired: 7 in]
            }
          }
          n250 = Unbundle By Name(w587) -> ("status"=w601:bool)
          n251 = local read "Scan"() -> (w599:bool)
          n252 = Compound Arithmetic op=OR(w601, w599) -> (w600:bool)
        }
      }
      frame True {
        n253 = local read "Step X"() -> (w621:dbl)
        n254 = local read "Travel per Pulse (mm)"() -> (w620:dbl)
        n255 = local read "Cur. Pos Y"() -> (w631:dbl)
        n256 = call "Sigma_TriggerOut.vi"("Axis(1)"=1, "error in (no error)"=w622, "Trigger distance (mm)"=w621, "Travel per Pulse (mm)"=w620, "VISA resource name"=w625) -> ("error out"=w623:errorcluster, "VISA resource name out"=w624:refnum<visa-resource-name>)  [unwired: 5 in]
        n257 = while {
          shift-right: [w651] -> _
          shift-left: TRUE ("Direction (+)") -> [w664]
          tunnel: w631 -> [w663]
          tunnel: [w659] -> w630
          tunnel: w624 -> [w666]
          tunnel: w623 -> [w665]
          tunnel: [w652] -> w628
          tunnel: [w649] -> w627
          tunnel: w620 -> [w640]
          stop <- w659 stop-if-true
          # "5. Stop scan condition"
          # "3. Run Step Y"
          # "2. wait until run to X-length"
          # "1. Move in X axis\n    Invert direction after moved Step Y"
          # "4. Update Y Possition"
          n258 = flat-sequence {
            tunnel: w666 -> [w672]
            tunnel: w665 -> [w671]
            tunnel: w664 -> [w677]
            tunnel: w663 -> [w675]
            tunnel: [w676] -> w639
            tunnel: [w670] -> w637
            tunnel: [w669] -> w635
            tunnel: [w675] -> w633
            tunnel: w640 -> [w668]
            tunnel: w639 -> [w682]
            tunnel: [w682] -> w638
            tunnel: w637 -> [w681]
            tunnel: [w681] -> w636
            tunnel: w635 -> [w680]
            tunnel: [w680] -> w634
            tunnel: w633 -> [w679]
            tunnel: [w679] -> w632
            tunnel: w638 -> [w685]
            tunnel: w636 -> [w690]
            tunnel: w634 -> [w689]
            tunnel: w632 -> [w686]
            tunnel: [w688] -> w658
            tunnel: [w687] -> w657
            tunnel: [w686] -> w653
            tunnel: [w685] -> w651
            tunnel: [w738] -> w648
            tunnel: w658 -> [w738]
            tunnel: [w737] -> w646
            tunnel: w657 -> [w737]
            tunnel: [w736] -> w644
            tunnel: w653 -> [w736]
            tunnel: w648 -> [w746]
            tunnel: [w746] -> w647
            tunnel: w646 -> [w745]
            tunnel: [w745] -> w645
            tunnel: w644 -> [w740]
            tunnel: [w741] -> w643
            tunnel: [w756] -> w662
            tunnel: [w755] -> w661
            tunnel: w647 -> [w752]
            tunnel: w645 -> [w751]
            tunnel: w643 -> [w748]
            tunnel: w662 -> [w770]
            tunnel: w661 -> [w769]
            tunnel: [w768] -> w654
            tunnel: [w767] -> w650
            tunnel: [w819] -> w656
            tunnel: [w818] -> w655
            tunnel: w654 -> [w818]
            tunnel: w650 -> [w819]
            tunnel: [w817] -> w641
            tunnel: w656 -> [w832]
            tunnel: [w833] -> w649
            tunnel: w655 -> [w833]
            tunnel: [w832] -> w652
            tunnel: [w831] -> w642
            tunnel: w641 -> [w831]
            frame #0 {
              n259 = local read "X-length"() -> (w674:dbl)
              n260 = local write "Move X"(FALSE ("Move X")) -> ()
              n261 = Not(x=w677) -> (.not. x?=w676:bool)
              n262 = call "Sigma_MoveAbs.vi"("Direction (+)"=w676, "Axis (1)"=1, "error in (no error)"=w671, "Travel (1mm)"=w674, "Travel per Pulse (0.004mm)"=w668, "VISA resource name"=w672) -> ("error out"=w669:errorcluster, "VISA resource name out"=w670:refnum<visa-resource-name>)  [unwired: 4 in]
            }
            frame #1 {
              n263 = Wait (ms)(milliseconds to wait=10.0 ("y")) -> ()  [unwired: 1 out]
            }
            frame #2 {
              n264 = local read "Cur. Pos X"() -> (w683:dbl)
              n265 = local read "Cur. Pos Y"() -> (w684:dbl)
              n266 = while {
                tunnel: w690 -> [w703]
                tunnel: w689 -> [w704]
                tunnel: [w702] -> w688
                tunnel: [w701] -> w687
                shift-right: [w695] -> _
                shift-left: w684 -> [w694]
                shift-right: [w696] -> _
                shift-left: w683 -> [w693]
                tunnel: w683 -> [w692]
                stop <- w711 stop-if-true
                # "Stop at LS"
                # "Send command and get position"
                n267 = local read "Travel per Pulse (mm)"() -> (w707:dbl)
                n268 = local read "X-length"() -> (w699:dbl)
                n269 = Wait Until Next ms Multiple(millisecond multiple=u32 100) -> ()  [unwired: 1 out]
                n270 = call "Sigma_GetPos.vi"("VISA resource name"=w703, "Travel per Pulse (mm)"=w707, "Init Pos X (mm)"=w693, "Init  Pos Y (mm)"=w694, "error in (no error)"=w704) -> ("Pos X (mm)"=w696:dbl, "Pos Y (mm)"=w695:dbl, "VISA resource name out"=w706:refnum<visa-resource-name>, "State String"=w708:string, "error out"=w705:errorcluster)  [unwired: 6 in]
                n271 = Subtract(x=w692, y=w696) -> (x-y=w698:dbl)
                n272 = local write "Cur. Pos X"(w696) -> ()
                n273 = local write "Cur. Pos Y"(w695) -> ()
                n274 = local write "Move X"(TRUE ("Move X")) -> ()
                n275 = Absolute Value(x=w698) -> (abs(x)=w700:dbl)
                n276 = Greater Or Equal?(x=w700, y=w699) -> (x >= y?=w697:bool)
                n277 = local read "Stop Scan"() -> (w710:bool)
                n278 = case shown="\"K\", Default" w708 {
                  tunnel: [w714 w719 w724 w729] -> w702
                  tunnel: [w713 w718 w723 w728] -> w701
                  tunnel: w706 -> [w714 w716 w721 w726]
                  tunnel: w705 -> [w713 w715 w720 w725]
                  frame "K", Default {
                  }
                  frame "L" {
                    n279 = call "Sigma_Stop.vi"("Axis (1)"="1", "error in (no error)"=w715, "VISA resource name"=w716) -> ("error out"=w718:errorcluster, "VISA resource name out"=w719:refnum<visa-resource-name>)  [unwired: 7 in]
                  }
                  frame "M" {
                    n280 = call "Sigma_Stop.vi"("Axis (1)"="2", "error in (no error)"=w720, "VISA resource name"=w721) -> ("error out"=w723:errorcluster, "VISA resource name out"=w724:refnum<visa-resource-name>)  [unwired: 7 in]
                  }
                  frame "W" {
                    n281 = call "Sigma_Stop.vi"("Axis (1)"="W", "error in (no error)"=w725, "VISA resource name"=w726) -> ("error out"=w728:errorcluster, "VISA resource name out"=w729:refnum<visa-resource-name>)  [unwired: 7 in]
                  }
                }
                n282 = Unbundle By Name(w701) -> ("status"=w712:bool)
                n283 = Compound Arithmetic op=OR(w712, w710, w697) -> (w711:bool)
              }
            }
            frame #3 {
              n284 = local read "1 Rate"() -> (w734:dbl)
              n285 = local read "Travel per Pulse (mm)"() -> (w735:dbl)
              n286 = local write "Move X"(FALSE ("Move X")) -> ()
              n287 = Divide(x=w734, y=w735) -> (x/y=w731:dbl)
              n288 = Add(x=w731, y=100.0) -> (x+y=w733:dbl)
              n289 = Wait (ms)(milliseconds to wait=w733) -> ()  [unwired: 1 out]
            }
            frame #4 {
              n290 = local read "Y-length"() -> (w739:dbl)
              n291 = local read "Cur. Pos Y"() -> (w744:dbl)
              n292 = Subtract(x=w744, y=w740) -> (x-y=w743:dbl)
              n293 = Absolute Value(x=w743) -> (abs(x)=w742:dbl)
              n294 = Greater Or Equal?(x=w742, y=w739) -> (x >= y?=w741:bool)
            }
            frame #5 {
              # "Stop Y"
              n295 = local read "Step Y"() -> (w754:dbl)
              n296 = local read "Y-length"() -> (w753:dbl)
              n297 = local read "Stop Scan"() -> (w750:bool)
              n298 = Greater Or Equal?(x=w754, y=w753) -> (x >= y?=w749:bool)
              n299 = Compound Arithmetic op=OR(w748, w749, w750) -> (w747:bool)
              n300 = case shown="False" w747 {
                tunnel: [w761 w766] -> w756
                tunnel: [w760 w765] -> w755
                tunnel: w752 -> [w758 w766]
                tunnel: w751 -> [w757 w765]
                frame False {
                  n301 = local read "Travel per Pulse (mm)"() -> (w759:dbl)
                  n302 = local read "Step Y"() -> (w763:dbl)
                  n303 = call "Sigma_MoveAbs.vi"("Axis (1)"=2, "error in (no error)"=w757, "Travel (1mm)"=w763, "Travel per Pulse (0.004mm)"=w759, "VISA resource name"=w758) -> ("error out"=w760:errorcluster, "VISA resource name out"=w761:refnum<visa-resource-name>)  [unwired: 5 in]
                }
                frame True {
                  n304 = local write "Stop Scan"(TRUE ("Stop Scan")) -> ()
                }
              }
            }
            frame #6 {
              n305 = disable-structure shown="Disabled" {
                disable-tunnel: w770 -> [w776 w816]
                disable-tunnel: w769 -> [w775 w815]
                disable-tunnel: [w774 w815] -> w768
                disable-tunnel: [w773 w816] -> w767
                frame Disabled {
                  n306 = local read item#-1() -> (w772)
                  n307 = local read item#-1() -> (w771)
                  n308 = while {
                    tunnel: w776 -> [w788]
                    tunnel: w775 -> [w789]
                    tunnel: [w787] -> w773
                    tunnel: [w786] -> w774
                    shift-right: [w781] -> _
                    shift-left: w771 -> [w778]
                    shift-right: [w780] -> _
                    shift-left: w772 -> [w779]
                    tunnel: w771 -> [w777]
                    stop <- w796 stop-if-true
                    # "Stop at LS"
                    # "Send command and get position"
                    n309 = local read item#-1() -> (w792)
                    n310 = Wait Until Next ms Multiple(millisecond multiple=u32 100) -> ()  [unwired: 1 out]
                    n311 = local read item#-1() -> (w784)
                    n312 = call "Sigma_GetPos.vi"("VISA resource name"=w788, "Travel per Pulse (mm)"=w792, "Init Pos X (mm)"=w779, "Init  Pos Y (mm)"=w778, "error in (no error)"=w789) -> ("Pos X (mm)"=w780:dbl, "Pos Y (mm)"=w781:dbl, "VISA resource name out"=w791:refnum<visa-resource-name>, "State String"=w793:string, "error out"=w790:errorcluster)  [unwired: 6 in]
                    n313 = Subtract(x=w777, y=w781) -> (x-y=w783:dbl)
                    n314 = local write item#-1(w780) -> ()
                    n315 = local write item#-1(w781) -> ()
                    n316 = Absolute Value(x=w783) -> (abs(x)=w785:dbl)
                    n317 = Greater Or Equal?(x=w785, y=w784) -> (x >= y?=w782:bool)
                    n318 = local read "Stop Scan 2"() -> (w795:bool)
                    n319 = case shown="\"K\", Default" w793 {
                      tunnel: [w799 w804 w809 w814] -> w787
                      tunnel: [w798 w803 w808 w813] -> w786
                      tunnel: w791 -> [w799 w801 w806 w811]
                      tunnel: w790 -> [w798 w800 w805 w810]
                      frame "K", Default {
                      }
                      frame "L" {
                        n320 = call "Sigma_Stop.vi"("Axis (1)"="1", "error in (no error)"=w800, "VISA resource name"=w801) -> ("error out"=w803:errorcluster, "VISA resource name out"=w804:refnum<visa-resource-name>)  [unwired: 7 in]
                      }
                      frame "M" {
                        n321 = call "Sigma_Stop.vi"("Axis (1)"="2", "error in (no error)"=w805, "VISA resource name"=w806) -> ("error out"=w808:errorcluster, "VISA resource name out"=w809:refnum<visa-resource-name>)  [unwired: 7 in]
                      }
                      frame "W" {
                        n322 = call "Sigma_Stop.vi"("Axis (1)"="W", "error in (no error)"=w810, "VISA resource name"=w811) -> ("error out"=w813:errorcluster, "VISA resource name out"=w814:refnum<visa-resource-name>)  [unwired: 7 in]
                      }
                    }
                    n323 = Unbundle By Name(w786) -> ("status"=w797:bool)
                    n324 = Compound Arithmetic op=OR(w797, w795, w782) -> (w796:bool)
                  }
                }
                frame Enabled {
                }
              }
            }
            frame #7 {
              n325 = local read "Stop Scan"() -> (w817:bool)
            }
            frame #8 {
              # "waiting for stop speed\naxis 2 + 100ms more"
              n326 = local read "2 Rate"() -> (w823:dbl)
              n327 = local read "Travel per Pulse (mm)"() -> (w822:dbl)
              n328 = local read "Step Y"() -> (w830:dbl)
              n329 = local read "2 Max"() -> (w829:dbl)
              n330 = Compound Arithmetic op=MULTIPLY(w823, invert w822, 2.0 ("value")) -> (w820:dbl)
              n331 = Compound Arithmetic op=MULTIPLY(w830, invert w829, 1000.0 ("value")) -> (w827:dbl)
              n332 = Add(x=w820, y=w827) -> (x+y=w826:dbl)
              n333 = Add(x=w826, y=100.0) -> (x+y=w824:dbl)
              n334 = Wait (ms)(milliseconds to wait=w824) -> ()  [unwired: 1 out]
            }
          }
          n335 = Unbundle By Name(w649) -> ("status"=w660:bool)
          n336 = Compound Arithmetic op=OR(w660, w642) -> (w659:bool)
        }
        "Move X" <- w626
      }
    }
  }
  n337 = call <vilib>:"Simple Error Handler.vi"() -> ()  [unwired: 5 in, 5 out]
